vi "RealTimeAcq_SynthFoc_Rev1.vi"(4 "Frames/s":sgl=2.0, 5 "return to start":bool, 6 "Scan Axis":i8=3, 7 "Motion Board ID":T3=1 min=1 max=32 step=1, 8 "BKPT Shift":i32=75, 9 "mode":T1=enum."Full 25 Ch") -> (0 "error out":errorcluster, 2 "Bd ID Out":T2)   [LabVIEW 2022 SP3]
uses:
  ScanningControl/Motion Controllers/-MotionRoutines/MotionGlobals.vi
  <vilib>/Motion/FlexMotion/FunctionsVIs/Trajectory.llb/Load Acceleration/Deceleration.flx
  <vilib>/Motion/FlexMotion/CustomControls/CustomControls.llb/Axis To Control.flx
  <vilib>/Motion/FlexMotion/CustomControls/CustomControls.llb/Program.flx
  <instrlib>/niScope/Acquire/Fetch/niScope Multi Fetch Binary 8.vi
  <vilib>/Platform/TimedLoop/XDataNode/XDataNode.xnode
  <vilib>/Platform/TimedLoop/XDataNode/nitl_modes.ctl
  <vilib>/Platform/TimedLoop/XDataNode/XDNodeRunTimeDep.lvlib
  <vilib>/Platform/TimedLoop/XDataNode/wakeup.ctl
  <vilib>/Platform/TimedLoop/XDataNode/timing_clust.ctl
  <vilib>/Motion/FlexMotion/FunctionsVIs/Trajectory.llb/Wait for Move Complete (8 axes).flx
  <instrlib>/Acqiris Dx/Acqiris Dx.lvlib
  Annular Array/-SynthApperture/TimeShiftDataI8.vi
  <vilib>/DAQmx/write.llb/DAQmx Write (Digital 1D Bool NChan 1Samp 1Line).vi
  <vilib>/Analysis/NI_AALBase.lvlib
  <vilib>/Analysis/baseanly.llb/Mean (DBL).vi
  Real Time/-RT_support/RealTimeMode.ctl
panel:
  in  "Velocity Scale (%)":i16(slide) scale=50.0..110.0
  in  "Raw Name":string="raw"
  in  "Save Raw":bool
  in  "Type of Mean":u16(ring) items=["Mean from lines", "Mean just lines", "Poly Mean", "No mean"]
  out "Display queue":i32
  out "SF queue":i32
  out "Record queue":i32
  out "Display index":i32
  out "Read Loop":i32
  out "Read Data index":i32
  in  "Round to ROC?":bool
  in  "F3 20 MHz":dbl[](array[numeric])=[0.0, 0.0021173000000000003, 0.002217038688303391, 0.003063649156506908, 0.0031631091439381287, 0.0038030513383040436, 0.003902223261134889, 0.004435332245982045, 0.004534208485358321, 0.004999044189180914]
  in  "F2 40MHz":sgl[](array[numeric])=[0.0, 0.00132, 0.00142, 0.0019, 0.002, 0.00236, 0.00245, 0.00275, 0.00285, 0.0031]
  in  "One Way Receive":bool
  out "SF Index":i32
  in  "stop out":bool
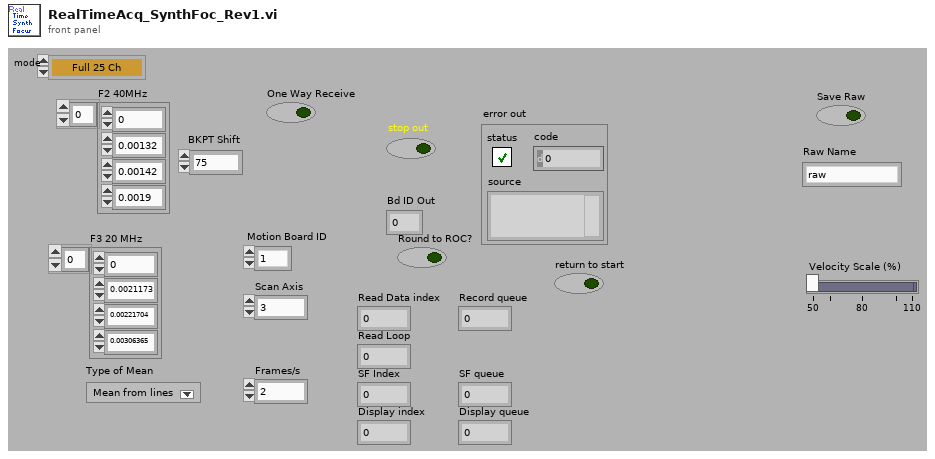
[diagram p1: front panel]
types:
  T1 = typedef "RealTimeMode.ctl" = enum16{"1T/5R", "1T/5R Deep Mem", "Full 25 Ch", "Drop Ch 5", "Drop Ch 5,4", "Drop Ch 5,4,3", "Drop Ch 5,4,3,2", "All 25 FIFO CH by CH", "Line by line 2 Ch", "Line by line All", "Deep Memory 2 CH", "Drop Ch 5 (3 Trig)", "test", "Drop Ch 5 XMIT", "Drop Ch 5,4 XMIT", "Drop Ch 5,4,3 XMIT"}
  T2 = typedef "Bd Id Out" = u8
  T3 = typedef "Board Id" = u8
  T4 = typedef "location.ctl" = enum16{"Automatic", "WCM Main", "Hawaii", "Columbia MM3000", "Columbia  NI System", "NYU", "RRI 2", "UHI Allen", "CUMC RT", "Chiba", "Stony Brook", "WCM Microscopy", "WCM Aeoretch", "WCM Optics Lab", "WCM Main 2Axis", "WCM Rotation", "WCM SAM SMAC", "SERI GP"}
  T5 = typedef "Program.flx" = u8
  T6 = typedef "XDNodeRunTimeDep.lvlib/timing_clust.ctl" = cluster{"Expected End [f-1]":u64, "Actual End [f-1]":u64, "Finished Late? [f-1]":bool, "Expected End [i-1]":u64, "Actual End [i-1]":u64, "Finished Late? [i-1]":bool, "Expected Start [i]":u64, "Actual Start [i]":u64, "Expected Start [f]":u64, "Actual Start [f]":u64, "Source Name":string, "Structure Name":string, "Period":i64, "Deadline":i64, "Offset":i64, "Start":i64, "Priority":i32, "Timeout":i32, "Mode":T7, "Wakeup Reason":T8, "Error":errorcluster, "Source Type":string, "Secondary Source Type":string, "Global End Time":u64, "Global Start Time":u64, "Frame Duration":u64, "Iteration Duration":u64, "Assigned CPU":i32, "I/O Scan Engine Mode":u32}
  T7 = typedef "XDNodeRunTimeDep.lvlib/nitl_modes.ctl" = enum32{"No Change", "Process missed periods, maintain original phase", "Discard missed periods, maintain original phase", "Process missed periods, ignore original phase", "Discard missed periods, ignore original phase"}
  T8 = typedef "XDNodeRunTimeDep.lvlib/wakeup.ctl" = enum32{"Normal", "Aborted", "Asynchronous wakeup", "Timing source error", "Timed loop error", "Timeout"}
  T9 = cluster{"gain":dbl, "wfm":i8[][], bool, "max queue size (-1, unlimited)":i32}
  T10 = typedef "Axis To Control.flx" = u16
  T11 = cluster{"ZoneStart":sgl[], "ZoneShift":sgl[], "ZoneLength":sgl[]}
  T12 = cluster{"ZoneStart":sgl[], "ZoneShift":sgl[], "ZoneLength":sgl[]}[][]
  T13 = cluster{"ZoneStart":sgl[], "ZoneShift":sgl[], "ZoneLength":sgl[]}[]
  T14 = cluster{"actualSamples":i32, "absoluteInitialX":dbl, "relativeInitialX":dbl, "xIncrement":dbl, "offset":dbl, "gain":dbl, "reserved1":dbl, "reserved2":dbl}[]
  T15 = cluster{"actualSamples":i32, "absoluteInitialX":dbl, "relativeInitialX":dbl, "xIncrement":dbl, "offset":dbl, "gain":dbl, "reserved1":dbl, "reserved2":dbl}
  T16 = cluster{"gain":dbl, "wfm":i8[][], "Reverse?":bool, i32}
  T17 = cluster{"dig gain":dbl, "Array":i8[][], "Reverse?":bool}
  T18 = typedef "Resource Out (Enum).flx" = u16
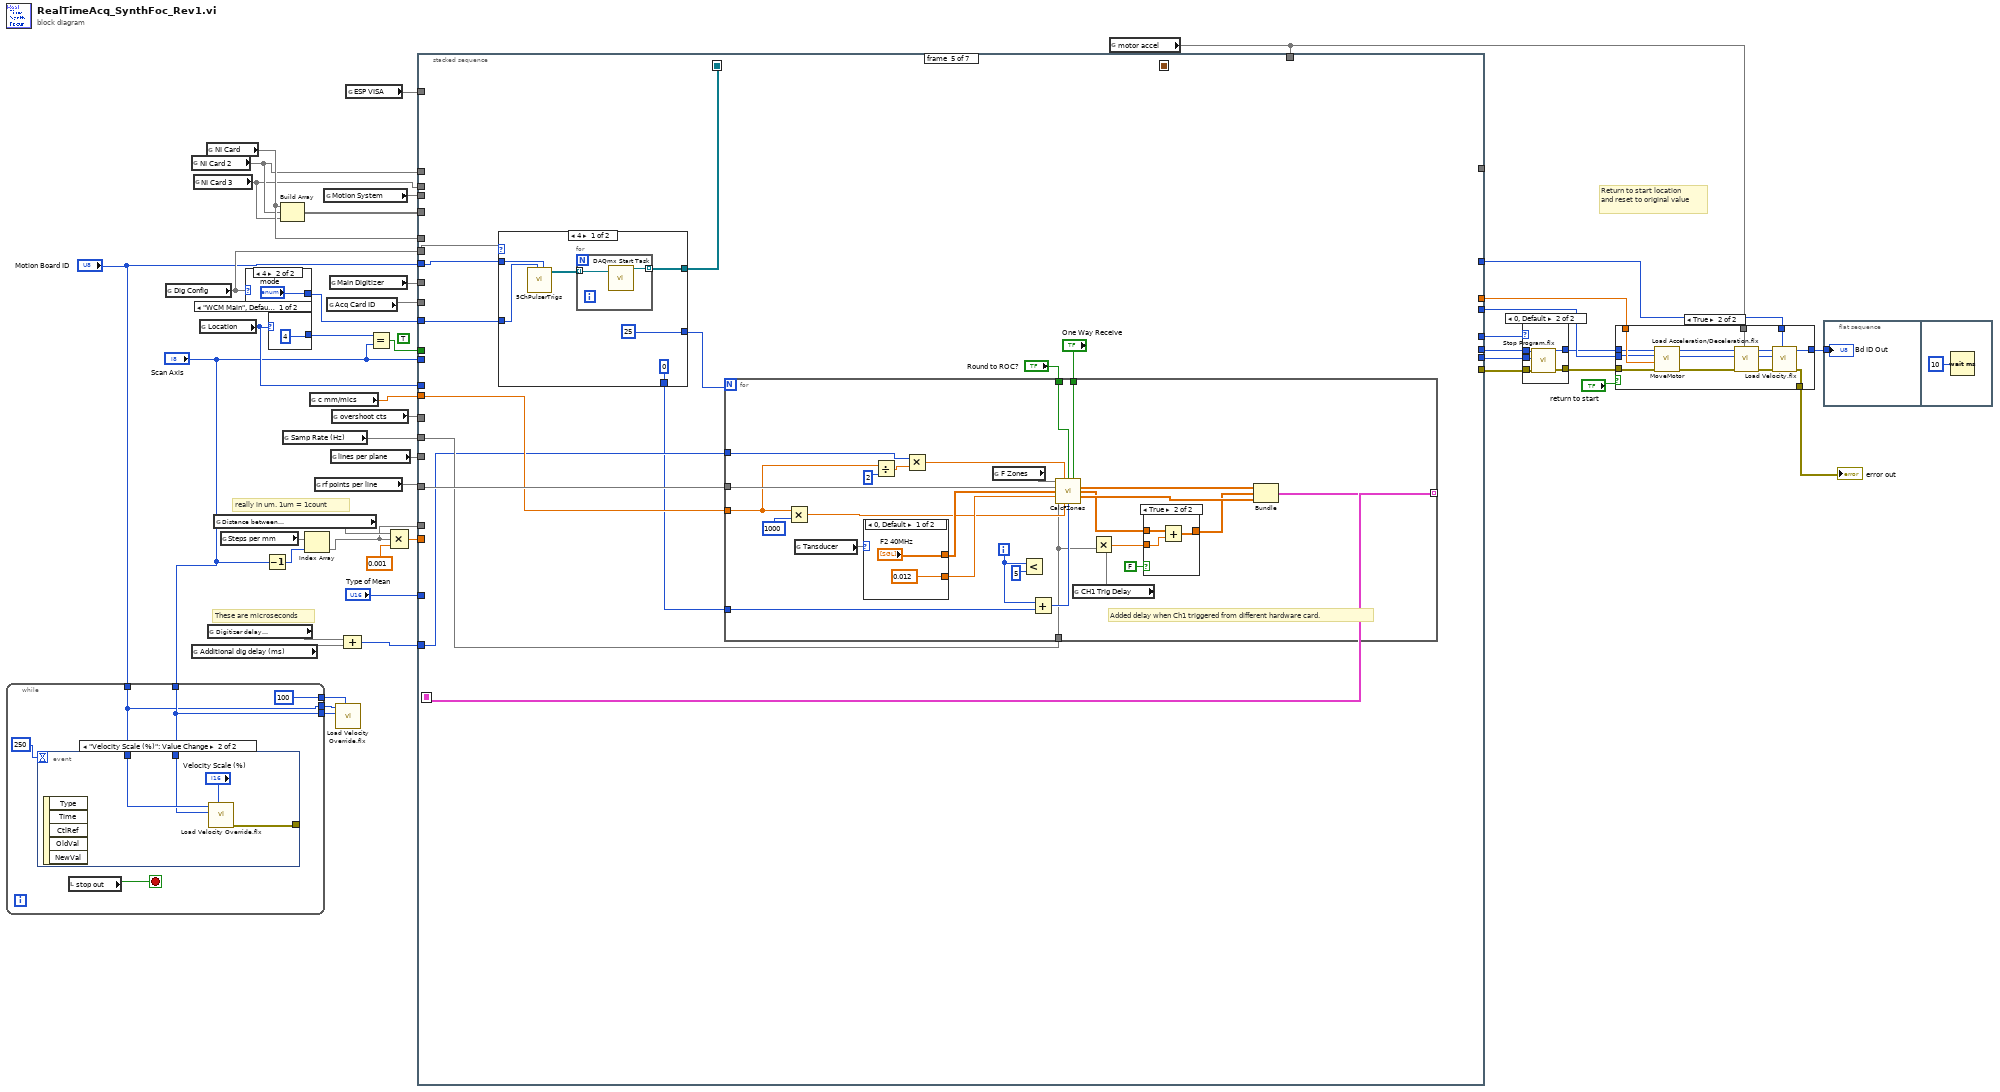
[diagram p0: block diagram]
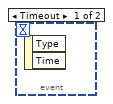
[diagram p2: hidden frame]
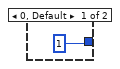
[diagram p3: hidden frame]
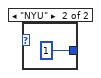
[diagram p6: hidden frame]
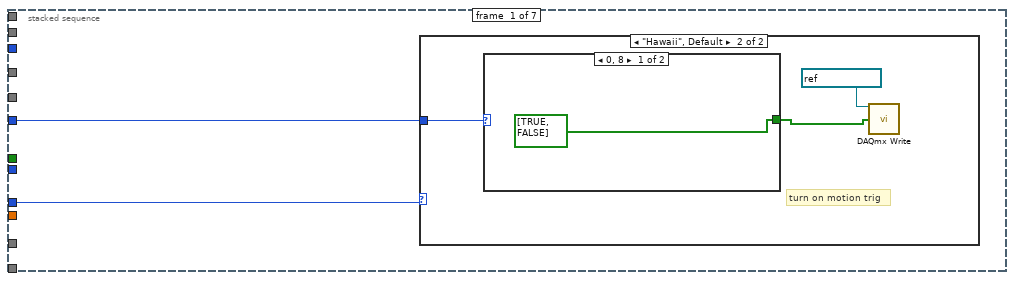
[diagram p7: hidden frame]
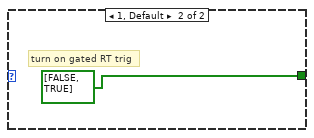
[diagram p9: hidden frame]
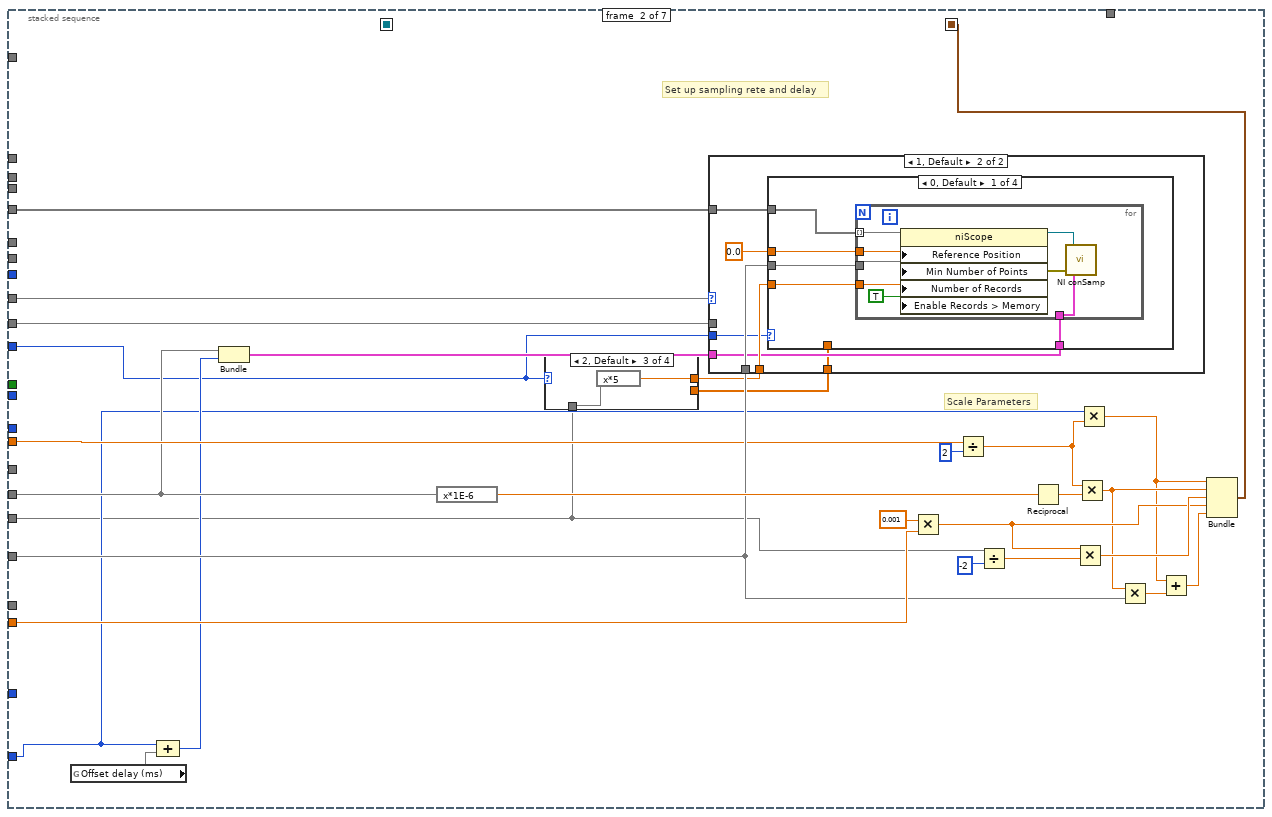
[diagram p10: hidden frame]
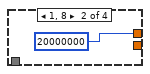
[diagram p12: hidden frame]
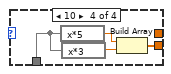
[diagram p13: hidden frame]
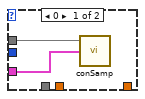
[diagram p14: hidden frame]
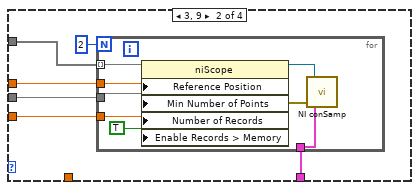
[diagram p15: hidden frame]
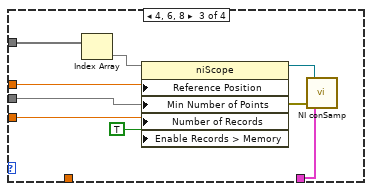
[diagram p16: hidden frame]
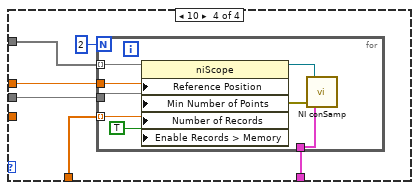
[diagram p17: hidden frame]
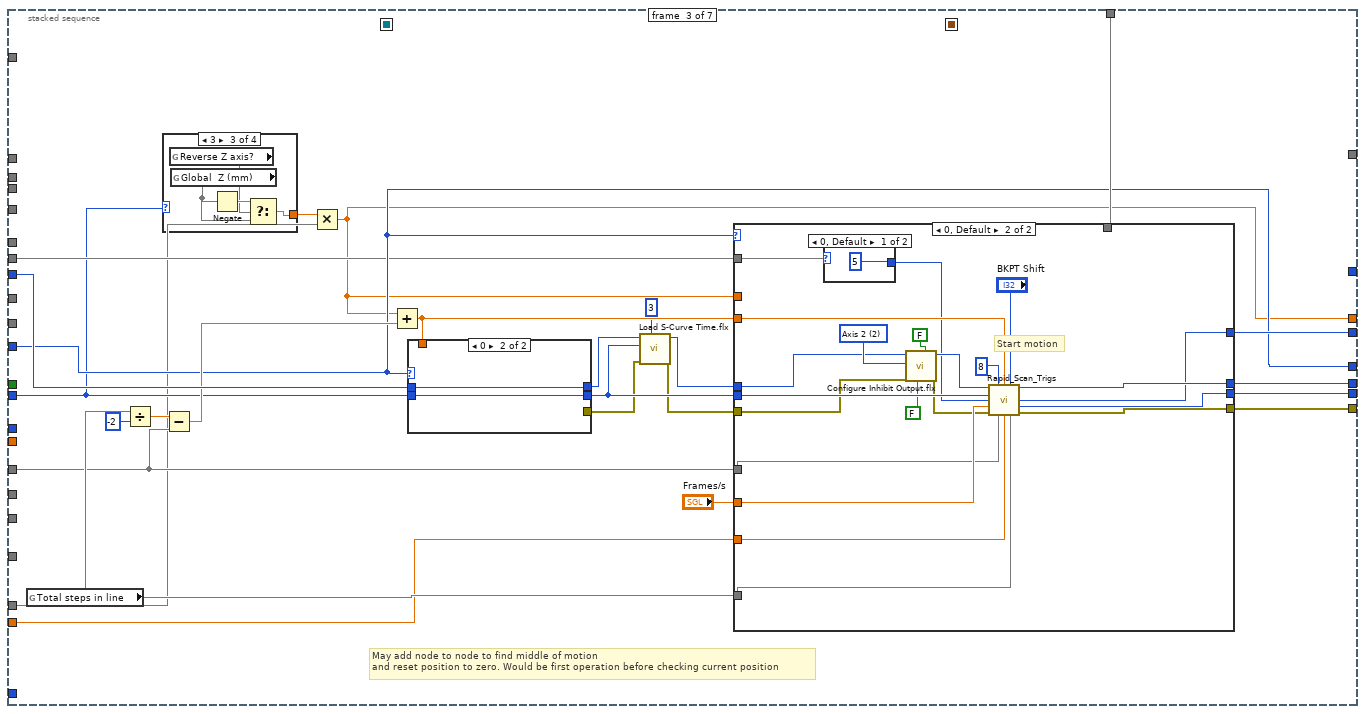
[diagram p18: hidden frame]
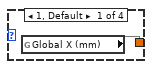
[diagram p19: hidden frame]
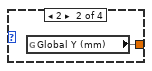
[diagram p20: hidden frame]
diagram:
  (unwired) TRUE
  # "These are microseconds"
  # "really in um. 1um = 1count"
  # "Return to start location and reset to original value"
  n1 = while {
    tunnel: "Motion Board ID" -> [w47]
    tunnel: "Scan Axis" -> [w48]
    tunnel: [100] -> w3
    tunnel: [w48] -> w2
    tunnel: [w47] -> w1
    stop <- w51 stop-if-true
    n2 = event shown="[1] \"Velocity Scale (%)\": Value Change" {
      selector: _ -> [_ _]
      dyn-events: _ -> [_ _]
      timeout: 250 -> [_ _]
      tunnel: w47 -> [_ w54]
      tunnel: w48 -> [_ w53]
      tunnel: [_ w52] -> _
      event Timeout {
        n3 = event-data() -> ()  [unwired: 1 in, 2 out]
      }
      event "Velocity Scale (%)": Value Change {
        n4 = event-data() -> ()  [unwired: 1 in, 5 out]
        n5 = call <vilib>:"Load Velocity Override.flx"("Override  Percentage (100%)"="Velocity Scale (%)", "Axis or Vector Space"=w53, "Board ID"=w54) -> ("error out"=w52:errorcluster)  [unwired: 4 in, 2 out]
      }
    }
    n6 = local read "stop out"() -> (w51:bool)
  }
  n7 = global read "MotionGlobals.vi" "Dig Config"() -> (w10)
  n8 = global read "MotionGlobals.vi" "NI Card 2"() -> (w14)
  n9 = global read "MotionGlobals.vi" "Additional dig delay (ms)"() -> (w25)
  n10 = global read "MotionGlobals.vi" "NI Card 3"() -> (w13)
  n11 = global read "MotionGlobals.vi" "Location"() -> (w28:T4)
  n12 = global read "MotionGlobals.vi" "NI Card"() -> (w15)
  n13 = global read "MotionGlobals.vi" "Digitizer delay\n (ms)"() -> (w26)
  n14 = global read "MotionGlobals.vi" "Distance between\nscan lines (mm)"() -> (w36)
  n15 = global read "MotionGlobals.vi" "Steps per mm"() -> (w9)
  n16 = case shown="4" w10 {
    tunnel: [i8 1 "mode"] -> w12
    frame 0, Default {
    }
    frame 4 {
    }
  }
  n17 = Decrement(x="Scan Axis") -> (x-1=w8:i8)
  n18 = case shown="\"WCM Main\", Default" w28 {
    tunnel: [i8 4 i8 1] -> w31
    frame "WCM Main", Default {
    }
    frame "NYU" {
    }
  }
  n19 = Build Array(w15, w14, w13) -> (w21:void[])
  n20 = global read "MotionGlobals.vi" "Samp Rate (Hz)"() -> (w23)
  n21 = Index Array(array=w9, index=w8) -> (element=w7)
  n22 = global read "MotionGlobals.vi" "c mm/mics"() -> (w27:sgl)
  n23 = global read "MotionGlobals.vi" "rf points per line"() -> (w45)
  n24 = global read "MotionGlobals.vi" "Motion System"() -> (w6)
  n25 = global read "MotionGlobals.vi" "Acq Card ID"() -> (w33)
  n26 = global read "MotionGlobals.vi" "Main Digitizer"() -> (w34)
  n27 = global read "MotionGlobals.vi" "lines per plane"() -> (w46)
  n28 = global read "MotionGlobals.vi" "overshoot cts"() -> (w44)
  n29 = call <vilib>:"Load Velocity Override.flx"("Override  Percentage (100%)"=w3, "Axis or Vector Space"=w2, "Board ID"=w1) -> ()  [unwired: 4 in, 3 out]
  n30 = Compound Arithmetic op=ADD(w26, w25) -> (w24:i32)
  n31 = global read "MotionGlobals.vi" "ESP VISA"() -> (w16)
  n32 = Equal?(x=w31, y="Scan Axis") -> (x = y?=w22:bool)
  n33 = Compound Arithmetic op=MULTIPLY(w36, w7, 0.001) -> (w35:dbl)
  n34 = global read "MotionGlobals.vi" "motor accel"() -> (w30)
  n35 = stacked-sequence {
    seq-local: [_ w87 _ _ _ _ _] -> [_ _ _ _ _ w312 _]
    seq-local: [_ _ _ _ w248 _ _] -> [_ _ _ _ _ w311 _]
    seq-local: [_ _ _ _ w245 _ _] -> [_ _ _ _ _ _ w2103]
    tunnel: w33 -> [_ w94 _ _ _ w320 _]
    tunnel: w46 -> [_ w69 _ _ _ w319 _]
    tunnel: [_ _ w187 _ _ _ _] -> w40
    tunnel: [_ _ w186 _ _ _ _] -> w42
    tunnel: w45 -> [_ w77 _ _ w254 w318 _]
    tunnel: [_ _ w184 _ _ _ _] -> w41
    tunnel: [_ _ w170 _ _ _ _] -> w39
    tunnel: w44 -> [_ _ w180 _ _ _ _]
    tunnel: [_ _ w183 _ _ _ _] -> w43
    tunnel: "Motion Board ID" -> [_ _ w179 w239 w244 w317 _]
    tunnel: [_ _ w174 _ _ _ _] -> w38
    tunnel: w12 -> [w60 w68 w174 _ w242 w307 w2104]
    tunnel: "Scan Axis" -> [_ _ w172 _ _ w308 _]
    tunnel: w35 -> [_ w80 w178 _ _ _ _]
    tunnel: w34 -> [_ w79 _ _ _ w316 _]
    tunnel: w15 -> [_ _ _ _ _ w315 _]
    tunnel: [_ _ _ _ _ w314 _] -> w32
    tunnel: w30 -> [_ _ w176 _ _ _ _]
    tunnel: w6 -> [_ _ _ w240 _ w313 _]
    tunnel: [_ _ _ _ _ w313 _] -> _
    tunnel: w28 -> [w61 _ _ _ _ w309 w2106]
    tunnel: w27 -> [_ w76 _ _ w253 _ _]
    tunnel: w24 -> [_ w72 _ _ w251 _ _]
    tunnel: w23 -> [_ w75 _ _ w252 _ _]
    tunnel: w22 -> [_ _ _ _ _ w306 _]
    tunnel: w21 -> [_ w71 _ _ _ w310 _]
    tunnel: w16 -> [_ _ _ _ _ _ _]
    tunnel: w14 -> [_ _ _ _ _ w305 _]
    tunnel: w13 -> [_ _ _ _ _ w304 _]
    tunnel: "Type of Mean" -> [_ _ _ _ _ w303 _]
    tunnel: w10 -> [_ _ w173 _ w243 _ _]
    tunnel: w7 -> [_ _ w169 _ _ _ _]
    frame #0 {
      n36 = case shown="\"Hawaii\", Default" w61 {
        tunnel: w60 -> [_ w64]
        frame "UHI Allen" {
        }
        frame "Hawaii", Default {
          # "turn on motion trig"
          n37 = case shown="0, 8" w64 {
            tunnel: [bool[] [TRUE, FALSE] ("data") bool[] [FALSE, TRUE] ("data")] -> w62
            frame 0, 8 {
            }
            frame 1, Default {
              # "turn on gated RT trig"
            }
          }
          n38 = call-poly <vilib>:"DAQmx Write.vi"("task/channels in"=refnum<k21> "DIO-L2 L3", "data"=w62) -> ()  [unwired: 11 in, 3 out]
        }
      }
    }
    frame #1 {
      # "Scale Parameters"
      # "Set up sampling rete and delay"
      n39 = global read "MotionGlobals.vi" "Offset delay (ms)"() -> (w74)
      n40 = Compound Arithmetic op=ADD(w72, w74) -> (w73:i32)
      n41 = Bundle("Samp Rate (Hz)"=w75, w73) -> (w95:cluster{"Samp Rate (Hz)":void, i32})  [unwired: 1 out]
      n42 = expression code="x*1E-6"(w75) -> (w78:dbl)
      n43 = case shown="2, Default" w68 {
        tunnel: [w96 20000000 w98 _] -> w70
        tunnel: w69 -> [w96 _ w99 w103]
        tunnel: [_ _ _ w100] -> w67
        frame 0 {
        }
        frame 1, 8 {
        }
        frame 2, Default {
          n44 = expression code="x*5"(w99) -> (w98:dbl)
        }
        frame 10 {
          n45 = expression code="x*5"(w103) -> (w102:dbl)
          n46 = expression code="x*3"(w103) -> (w101:dbl)
          n47 = Build Array(w102, w101) -> (w100:dbl[])
        }
      }
      n48 = case shown="1, Default" w79 {
        tunnel: w95 -> [w105 w110]
        tunnel: w94 -> [w104 _]
        tunnel: w77 -> [_ w111]
        tunnel: w70 -> [_ w112]
        tunnel: w71 -> [_ w109]
        tunnel: w68 -> [_ w107]
        tunnel: w67 -> [_ w106]
        frame 0 {
          n49 = call "conSamp.vi"("Sampling"=w105, "InstrumentID"=w104) -> ()  [unwired: 1 in, 2 out]
        }
        frame 1, Default {
          n50 = case shown="0, Default" w107 {
            tunnel: w112 -> [w117 w131 w148 _]
            tunnel: w111 -> [w116 w130 w147 w154]
            tunnel: w110 -> [w115 w129 w146 w153]
            tunnel: w109 -> [w114 w128 w144 w152]
            tunnel: 0.0 -> [w113 w127 w145 w151]
            tunnel: w106 -> [_ _ _ w149]
            frame 0, Default {
              n51 = for {
                tunnel: w117 -> [w120]
                tunnel: w116 -> [w125]
                tunnel: w114 -> [w122] mode=indexing
                tunnel: w115 -> [w121]
                tunnel: w113 -> [w119]
                n52 = property class="niScope"(reference=w122, "Reference Position"=w119, "Min Number of Points"=w125, "Number of Records"=w120, "Enable Records > Memory"=TRUE) -> (reference out=w124:refnum<k15>, error out=w123:errorcluster)  [unwired: 1 in]
                n53 = call "NI conSamp.vi"("error in"=w123, "Sampling"=w121, "InstrumentID"=w124) -> ()  [unwired: 2 out]
              }
            }
            frame 3, 9 {
              n54 = for {
                N: 2 -> [_]
                tunnel: w131 -> [w134]
                tunnel: w130 -> [w139]
                tunnel: w128 -> [w136] mode=indexing
                tunnel: w129 -> [w135]
                tunnel: w127 -> [w133]
                n55 = property class="niScope"(reference=w136, "Reference Position"=w133, "Min Number of Points"=w139, "Number of Records"=w134, "Enable Records > Memory"=TRUE) -> (reference out=w138:refnum<k15>, error out=w137:errorcluster)  [unwired: 1 in]
                n56 = call "NI conSamp.vi"("error in"=w137, "Sampling"=w135, "InstrumentID"=w138) -> ()  [unwired: 2 out]
              }
            }
            frame 4, 6, 8 {
              n57 = Index Array(array=w144) -> (element=w140)  [unwired: 1 in]
              n58 = property class="niScope"(reference=w140, "Reference Position"=w145, "Min Number of Points"=w147, "Number of Records"=w148, "Enable Records > Memory"=TRUE) -> (reference out=w143:refnum<k15>, error out=w142:errorcluster)  [unwired: 1 in]
              n59 = call "NI conSamp.vi"("error in"=w142, "Sampling"=w146, "InstrumentID"=w143) -> ()  [unwired: 2 out]
            }
            frame 10 {
              n60 = for {
                N: 2 -> [_]
                tunnel: w149 -> [w157] mode=indexing
                tunnel: w154 -> [w162]
                tunnel: w152 -> [w159] mode=indexing
                tunnel: w153 -> [w158]
                tunnel: w151 -> [w156]
                n61 = property class="niScope"(reference=w159, "Reference Position"=w156, "Min Number of Points"=w162, "Number of Records"=w157, "Enable Records > Memory"=TRUE) -> (reference out=w161:refnum<k15>, error out=w160:errorcluster)  [unwired: 1 in]
                n62 = call "NI conSamp.vi"("error in"=w160, "Sampling"=w158, "InstrumentID"=w161) -> ()  [unwired: 2 out]
              }
            }
          }
        }
      }
      n63 = Multiply(x=0.001, y=w80) -> (x*y=w85:dbl)
      n64 = Divide(x=w76, y=2) -> (x/y=w88:sgl)
      n65 = Divide(x=w69, y=-2) -> (x/y=w90:dbl)
      n66 = Reciprocal(x=w78) -> (1/x=w93:dbl)
      n67 = Multiply(x=w85, y=w90) -> (x*y=w86:dbl)
      n68 = Multiply(x=w88, y=w93) -> (x*y=w84:dbl)
      n69 = Multiply(x=w72, y=w88) -> (x*y=w82:sgl)
      n70 = Multiply(x=w84, y=w77) -> (x*y=w83:dbl)
      n71 = Add(x=w82, y=w83) -> (x+y=w81:sgl)
      n72 = Bundle(w82, w84, w86, w85, w81) -> (w87:cluster{sgl, dbl, dbl, dbl, sgl})  [unwired: 1 out]
    }
    frame #2 {
      # "May add node to node to find middle of motion\nand reset position to zero. Would be first operation before checking current position"
      n73 = global read "MotionGlobals.vi" "Total steps in line"() -> (w182)
      n74 = Divide(x=w182, y=-2) -> (x/y=w181:dbl)
      n75 = case shown="3" w172 {
        tunnel: [w189 w190 w191 w195] -> w171
        frame 1, Default {
          n76 = global read "MotionGlobals.vi" "Global X (mm)"() -> (w189)
        }
        frame 2 {
          n77 = global read "MotionGlobals.vi" "Global Y (mm)"() -> (w190)
        }
        frame 3 {
          n78 = global read "MotionGlobals.vi" "Reverse Z axis?"() -> (w192)
          n79 = global read "MotionGlobals.vi" "Global  Z (mm)"() -> (w193)
          n80 = Negate(x=w193) -> (-x=w194:dbl)
          n81 = Select(t=w194, s=w192, f=w193) -> (s? t:f=w191:dbl)
        }
        frame 4 {
          n82 = global read "MotionGlobals.vi" "Global  Axis 4"() -> (w195)
        }
      }
      n83 = Subtract(x=w181, y=w180) -> (x-y=w177:dbl)
      n84 = Multiply(x=w171, y=w169) -> (x*y=w170:dbl)
      n85 = Add(x=w170, y=w177) -> (x+y=w175:dbl)
      n86 = case shown="0" w174 {
        tunnel: w179 -> [w201 w203]
        tunnel: w172 -> [w200 w202]
        tunnel: [w199 w203] -> w168
        tunnel: [w198 w202] -> w166
        tunnel: [w197 _] -> w164
        tunnel: w175 -> [w196 _]
        frame 1, Default {
          n87 = call "MoveMotor.vi"("Target Position (0)"=w196, "Axis or Vector Space"=w200, "Motion Bd ID"=w201) -> ("error out"=w197:errorcluster, "Resource Output"=w198:u16, "Bd ID Out"=w199:u8)  [unwired: 2 in, 4 out]
        }
        frame 0 {
        }
      }
      n88 = call <vilib>:"Load S-Curve Time.flx"("S Curve Time (1)"=u16 3, "error in (no error)"=w164, "Axis or Vector Space"=w166, "Board ID"=w168) -> ("error out"=w163:errorcluster, "Bd ID Out"=w167:T2)  [unwired: 3 in, 1 out]
      n89 = case shown="0, Default" w174 {
        tunnel: "Frames/s" -> [w213 w236]
        tunnel: [w204 w235] -> w187
        tunnel: [w215 w234] -> w186
        tunnel: [_ w233] -> w184
        tunnel: [w214 w232] -> w183
        tunnel: w182 -> [w211 w231]
        tunnel: w178 -> [_ w230]
        tunnel: w180 -> [_ w229]
        tunnel: w167 -> [w215 w219]
        tunnel: w166 -> [w214 w228]
        tunnel: w163 -> [w205 w218]
        tunnel: w175 -> [_ w227]
        tunnel: w170 -> [w212 _]
        tunnel: w176 -> [_ _]
        tunnel: w173 -> [_ w216]
        frame 1, 8 {
          w207 = T5 6 ("Program (1)")
          w210 = FALSE
          n90 = call "Modulo_Triggers.vi"("Motion Settings In"=w215, "Axis"=w214, "Reverse ?"=w210, "Program (1)"=w207, 7:w213, "error in (no error)"=w205, 12:w211, "Offset"=w212) -> ("error out"=w206:errorcluster)  [unwired: 1 in, 6 out]
          n91 = Increment(x=w207) -> (x+1=w208:T5)
          n92 = Not(x=w210) -> (.not. x?=w209:bool)
          n93 = call "Modulo_Triggers.vi"("Motion Settings In"=w215, "Axis"=w214, "Reverse ?"=w209, "Program (1)"=w208, 7:w213, "error in (no error)"=w206, 12:w211, "Offset"=w212) -> ("error out"=w204:errorcluster)  [unwired: 1 in, 6 out]
        }
        frame 0, Default {
          w222 = T10 2 items=["Axis 1"=1, "Axis 2"=2, "Axis 3"=3, "Axis 4"=4, "Axis 5"=5, "Axis 6"=6, "Axis 7"=7, "Axis 8"=8] ("Axis")
          # "Start motion"
          n94 = case shown="0, Default" w216 {
            tunnel: [u32 5 u32 5 ("EOL Delay (ms)")] -> w217
            frame 0, Default {
            }
            frame 2 {
            }
          }
          n95 = call <vilib>:"Configure Inhibit Output.flx"("Enable"=FALSE, "Polarity (Active Low)"=FALSE, "error in (no error)"=w218, "Axis"=w222, "Board ID"=w219) -> ("error out"=w225:errorcluster, "Bd ID Out"=w226:T2)  [unwired: 1 in, 4 out]
          n96 = call "Rapid_Scan_Trigs.vi"("Board ID"=w226, "Program (1)"=T5 8, "Start Position"=w227, "BKPT Shift"="BKPT Shift", "Scan Axis"=w228, "Pause?"=w217, "# frames/ s"=w236, "error in (no error)"=w225, "overshoot"=w229, "step interval"=w230, "Total Steps (one way)"=w231) -> ("Bd ID Out"=w234:u8, "Axis Resource out"=w232:u16, "Program ID"=w233:u8, "error out"=w235:errorcluster)  [unwired: 1 out]
        }
      }
    }
    frame #3 {
      n97 = case shown="0, Default" w240 {
        tunnel: w239 -> [w241 _]
        frame 0, Default {
          n98 = call "CheckLimStat.vi"("Motion Board ID"=w241) -> ()
        }
        frame 1, 7 {
        }
      }
    }
    frame #4 {
      n99 = case shown="4" w243 {
        tunnel: [25 5] -> w247
        tunnel: [u32 0 w263] -> w246
        tunnel: [w257 _] -> w245
        tunnel: w244 -> [w256 _]
        tunnel: w242 -> [w255 _]
        frame 4 {
          n100 = call "5ChPulserTrigs.vi"("Motion Board ID"=w256, "mode"=w255) -> ("5CH Pulser Tasks"=w258:refnum<k21>[])  [unwired: 7 in, 1 out]
          n101 = for {
            tunnel: w258 -> [w262] mode=indexing
            tunnel: [w261] -> w257 mode=indexing
            n102 = call <vilib>:"DAQmx Start Task.vi"("task/channels in"=w262) -> ("task out"=w261:refnum<k21>)  [unwired: 13 in, 1 out]
          }
        }
        frame 0, Default {
          n103 = global read "MotionGlobals.vi" "Switch T/R"() -> (w266)
          n104 = Decrement(x=w266) -> (x-1=w265:dbl)
          n105 = Multiply(x=w265, y=5) -> (x*y=w263:i32)
        }
      }
      n106 = for {
        N: w247 -> [_]
        tunnel: w254 -> [w287]
        tunnel: w253 -> [w280]
        tunnel: w252 -> [w274]
        tunnel: w251 -> [w286]
        tunnel: "One Way Receive" -> [w285]
        tunnel: "Round to ROC?" -> [w284]
        tunnel: [w282] -> w248 mode=indexing
        tunnel: w246 -> [w277]
        i -> [w276]
        # "Added delay when Ch1 triggered from different hardware card."
        n107 = Multiply(x=w280, y=1000) -> (x*y=w281:sgl)
        n108 = global read "MotionGlobals.vi" "Tansducer"() -> (w290)
        n109 = case shown="0, Default" w290 {
          tunnel: ["F2 40MHz" "F3 20 MHz"] -> w289
          tunnel: [0.012 ("ROC (mm)") 0.031 ("ROC (mm)")] -> w288
          frame 0, Default {
          }
          frame 1 {
          }
        }
        n110 = Divide(x=w280, y=2) -> (x/y=w293:sgl)
        n111 = Multiply(x=w286, y=w293) -> (x*y=w279:sgl)
        n112 = global read "MotionGlobals.vi" "F Zones"() -> (w292)
        n113 = Less?(x=w276, y=5) -> ()  [unwired: 1 out]
        n114 = Add(x=w276, y=w277) -> (x+y=w278:u32)
        n115 = call "CalcFZones.vi"("F- zones"=w292, "delay (mm)"=w279, "Round to ROC?"=w284, "One Way Receive"=w285, "# rf points per line"=w287, "Radii (m)"=w289, "ROC (m)"=w288, "Sampling Rate"=w274, "c (m/s)"=w281, "File index number"=w278) -> ("ZoneStart"=w272:sgl[], "ZoneShift"=w271:sgl[], "ZoneLength"=w283:sgl[])  [unwired: 3 out]
        n116 = global read "MotionGlobals.vi" "CH1 Trig Delay"() -> (w269)
        n117 = Multiply(x=w269, y=w274) -> (x*y=w273:dbl)
        n118 = case shown="True" FALSE {
          tunnel: w271 -> [w295 w297]
          tunnel: [w295 w298] -> w270
          tunnel: w273 -> [_ w296]
          frame False {
          }
          frame True {
            n119 = Add(x=w297, y=w296) -> (x+y=w298:sgl[])
          }
        }
        n120 = Bundle("ZoneStart"=w272, "ZoneShift"=w270, "ZoneLength"=w283) -> (w282:T11)  [unwired: 1 in]
      }
    }
    frame #5 {
      n121 = case shown="True" w306 {
        tunnel: w320 -> [w328 _]
        tunnel: w319 -> [w329 w424]
        tunnel: w318 -> [w330 w423]
        tunnel: w317 -> [w326 w425]
        tunnel: w312 -> [w325 w422]
        tunnel: w316 -> [w324 _]
        tunnel: w315 -> [w323 w417]
        tunnel: [w322 w426] -> w314
        tunnel: w313 -> [w321 _]
        tunnel: w311 -> [_ w421]
        tunnel: w307 -> [_ w420]
        tunnel: w310 -> [_ w419]
        tunnel: w309 -> [_ _]
        tunnel: w308 -> [_ w418]
        tunnel: w305 -> [_ w416]
        tunnel: w304 -> [_ w415]
        tunnel: w303 -> [_ w414]
        frame False {
          n122 = while {
            tunnel: w330 -> [w352]
            tunnel: w329 -> [w342]
            tunnel: w328 -> [w351]
            shift-right: [w350] -> _
            shift-left: TRUE -> [w334]
            tunnel: w326 -> [w349]
            tunnel: w325 -> [w345]
            tunnel: w324 -> [w343]
            tunnel: w323 -> [w341]
            tunnel: w321 -> [w335]
            i -> [w344]
            stop <- w348 stop-if-true
            # "Display data"
            # "Get data"
            # "This is slower version for heavier mass motors. Scan stop, read data, scan etc"
            n123 = Select(t="1", s=w334, f="2") -> (s? t:f=w331:string)
            n124 = Select(t=T5 6 ("Program (1)"), s=w334, f=T5 7 ("Program (1)")) -> (s? t:f=w338:T5)
            n125 = case shown="1, Default" w343 {
              tunnel: w352 -> [w362 w390]
              tunnel: w342 -> [w361 w389]
              tunnel: w351 -> [w375 _]
              tunnel: w349 -> [w374 w401]
              tunnel: [w373 w400] -> w347
              tunnel: w338 -> [w369 w399]
              tunnel: [w356 w391] -> w340
              tunnel: w341 -> [_ w393]
              tunnel: w334 -> [w358 w384]
              tunnel: [w359 w383] -> w339
              tunnel: w335 -> [_ _]
              tunnel: w331 -> [_ _]
              frame 0 {
                n126 = call <instrlib>:"Configure Memory Settings.vi"("Number of Samples (1000)"=w362, "Number of Segments (1)"=w361, "Instrument ID"=w375) -> ("error out"=w372:errorcluster, "dup Instrument ID"=w370:u32)  [unwired: 1 in, 2 out]
                n127 = call <instrlib>:"Start Acquisition.vi"("error in (no error)"=w372, "Instrument ID"=w370) -> ("error out"=w368:errorcluster, "dup Instrument ID"=w371:u32)  [unwired: 2 in]
                n128 = stacked-sequence {
                  tunnel: w368 -> [w382]
                  tunnel: [w382] -> w367
                  frame #0 {
                    n129 = Wait (ms)(milliseconds to wait=20) -> ()  [unwired: 1 out]
                  }
                }
                n130 = call <vilib>:"Run Program.flx"("error in (no error)"=w367, "Program (1)"=w369, "Board ID"=w374) -> ("error out"=w366:errorcluster, "Bd ID Out"=w373:T2)  [unwired: 4 out]
                n131 = stacked-sequence {
                  tunnel: w366 -> [w379]
                  tunnel: [w379] -> w365
                  frame #0 {
                    n132 = Wait (ms)(milliseconds to wait=20) -> ()  [unwired: 1 out]
                  }
                }
                n133 = call "WaitForSegs.vi"("Acqiris ID"=w371, "lines per plane"=w361, "error in"=w365, "Timeout"=5000) -> ("dup Instrument ID"=w364:u32, "error out"=w363:errorcluster)  [unwired: 2 out]
                n134 = call "GetWaveform.vi"("Acq ID Out"=w364, "Num Samps"=w362, "Num Segs"=w361, "error in"=w363) -> ("Acquired Waveform16 bit"=w360:i16[][], "error out"=w356:errorcluster)  [unwired: 2 in, 8 out]
                n135 = case shown="True" w358 {
                  tunnel: w360 -> [w376 w378]
                  tunnel: [w376 w377] -> w359
                  frame False {
                  }
                  frame True {
                    n136 = call "ReverseData.vi"("Array in"=w378) -> ("Array out"=w377:i16[][])
                  }
                }
              }
              frame 1, Default {
                w387 = u16 1 items=["Simple Read", "RT Read", "RT Save", "Scaled Voltage"] ("Read Method")
                n137 = property class="niScope"(reference=w393, "Number of Records"=w389, "Min Number of Points"=w390) -> (reference out=w395:refnum<k15>, error out=w394:errorcluster)  [unwired: 1 in]
                n138 = call <instrlib>:"niScope Initiate Acquisition.vi"("instrument handle"=w395, "error in"=w394) -> ("instrument handle out"=w388:refnum<k15>, "error out"=w398:errorcluster)  [unwired: 1 in, 11 out]
                n139 = stacked-sequence {
                  tunnel: w398 -> [w405]
                  tunnel: [w405] -> w397
                  frame #0 {
                    n140 = Wait (ms)(milliseconds to wait=u32 5) -> ()  [unwired: 1 out]
                  }
                }
                n141 = call <vilib>:"Run Program.flx"("error in (no error)"=w397, "Program (1)"=w399, "Board ID"=w401) -> ("error out"=w396:errorcluster, "Bd ID Out"=w400:T2)  [unwired: 4 out]
                n142 = stacked-sequence {
                  tunnel: w396 -> [w402]
                  tunnel: [w402] -> w392
                  frame #0 {
                    n143 = Wait (ms)(milliseconds to wait=u32 20) -> ()  [unwired: 1 out]
                  }
                }
                n144 = call "NI GetWaveform.vi"("Acq ID In"=w388, "Read Method"=w387, "timeout"=5.0, "Num Samps"=w390, "Reverse?"=w384, "Num Segs"=w389, "error in"=w392, "Channel"=1) -> ("Acquired Waveform16 bit"=w383:i8[][], "error out"=w391:errorcluster)  [unwired: 2 in, 4 out]
              }
            }
            n145 = case shown="No Error" w340 {
              selector: w340 -> [w407 w412]
              tunnel: [w408 w412] -> w346
              tunnel: [w411 TRUE] -> w348
              tunnel: w345 -> [w410 _]
              tunnel: w344 -> [w409 _]
              tunnel: w339 -> [w406 _]
              frame No Error {
                n146 = call "CurrentPlane.vi"("Axis Vals"=w410, "error in"=w407, "Frame"=w409, "Data"=w406) -> ("error out"=w408:errorcluster, "stop out"=w411:bool)  [unwired: 6 in]
              }
              frame Error {
              }
            }
            n147 = local write "SF Index"(w344) -> ()
            n148 = case shown="1, Default" w335 {
              tunnel: w347 -> [_ w355]
              tunnel: w346 -> [_ w354]
              tunnel: w338 -> [_ w353]
              frame 7 {
              }
              frame 1, Default {
                n149 = call <vilib>:"Stop Program.flx"("error in (no error)"=w354, "Program (1)"=w353, "Board ID"=w355) -> ()  [unwired: 6 out]
              }
            }
            n150 = Not(x=w334) -> (.not. x?=w350:bool)
          }
          n151 = global read "MotionGlobals.vi" "motor velocity"() -> (w322)
        }
        frame True {
          n152 = case shown="2" w420 {
            tunnel: [40000 40000 40000 40000 40000 40000 40000 40000 40000 40000 40000] -> w426
            tunnel: w425 -> [w452 w603 w757 w945 w1115 w1225 w1391 w1476 w1593 w1760 w1945]
            tunnel: w424 -> [w451 w599 w761 w927 w1111 w1229 w1392 w1477 w1558 w1742 w1921]
            tunnel: w423 -> [w450 w600 w738 w929 w1101 w1221 w1378 w1490 w1561 w1744 w1929]
            tunnel: w422 -> [w429 w568 w763 w950 w1120 w1231 w1397 w1484 w1578 w1765 w1950]
            tunnel: w421 -> [w445 w594 w771 w958 w1128 w1240 w1382 w1478 w1567 w1773 w1958]
            tunnel: w419 -> [w438 w577 _ _ _ _ _ w1471 _ _ _]
            tunnel: w418 -> [_ w579 _ _ _ _ _ _ w1586 _ _]
            tunnel: w417 -> [_ _ w749 w926 w1106 w1222 w1379 _ w1582 w1741 w1927]
            tunnel: w416 -> [_ _ w774 w924 _ w1243 _ _ _ w1739 w1925]
            tunnel: w415 -> [_ _ w773 _ _ w1242 _ _ _ _ _]
            tunnel: w414 -> [_ _ _ _ _ _ _ _ _ _ _]
            frame 0, Default {
              # "1T/5R flip flop version"
              n153 = Array To Cluster(array=w438) -> (cluster=w437:cluster{"[0]":void, "[1]":void, "[2]":void})
              n154 = Unbundle(w437) -> ("[0]"=w428, "[1]"=w436, "[2]"=w435)
              n155 = Obtain Queue(max queue size (-1, unlimited)=4, element data type=cluster{"gain":dbl, bool} {"gain"=0.0, TRUE}) -> (queue out=w460:refnum<queue>)  [unwired: 2 in, 3 out]
              n156 = Index Array(array=w445) -> (element=w442:T11)  [unwired: 1 in]
              n157 = Index Array(array=w445, index=1) -> (element=w441:T11)
              n158 = Index Array(array=w445, index=2) -> (element=w440:T11)
              n159 = Index Array(array=w445, index=3) -> (element=w443:T11)
              n160 = Index Array(array=w445, index=4) -> (element=w444:T11)
              n161 = Obtain Queue(max queue size (-1, unlimited)=20, element data type=i8[][] [] ("Array")) -> (queue out=w453:refnum<queue>)  [unwired: 2 in, 3 out]
              n162 = Obtain Queue(max queue size (-1, unlimited)=4, element data type=cluster{bool, "Array":i16[][]} {TRUE, "Array"=[]}) -> (queue out=w433:refnum<queue>)  [unwired: 3 in, 2 out]
              n163 = while {
                tunnel: w460 -> [w489]
                tunnel: [w520] -> w458
                tunnel: [w498] -> w457
                tunnel: w453 -> [w490]
                tunnel: w444 -> [w511]
                tunnel: w443 -> [w510]
                tunnel: w442 -> [w509]
                tunnel: w441 -> [w508]
                tunnel: w440 -> [w507]
                tunnel: [w485] -> w439
                tunnel: w433 -> [w502]
                i -> [w499]
                stop <- w520 stop-if-true
                w495 = 5000 ("timeout in ms (-1)")
                # "Dequeue data and synth focus"
                n164 = Dequeue Element(queue=w489, timeout in ms (-1)=w495) -> (queue out=w498:refnum<queue>, element=w519:cluster{"gain":dbl, bool}, error out=w497:errorcluster)  [unwired: 1 in, 1 out]
                n165 = Dequeue Element(queue=w490, timeout in ms (-1)=w495, error in (no error)=w497) -> (queue out=w488:refnum<queue>, element=w496:i8[][], error out=w494:errorcluster)  [unwired: 1 out]
                n166 = Unbundle(w519) -> (w501:bool)  [unwired: 1 out]
                n167 = call-poly "TimeShiftDataPoly.vi"("output cluster"=w509, "Array In"=w496) -> ("Array Out"=w482:i8[][])  [unwired: 1 in, 1 out]
                n168 = Dequeue Element(queue=w488, timeout in ms (-1)=w495, error in (no error)=w494) -> (queue out=w518:refnum<queue>, element=w515:i8[][], error out=w493:errorcluster)  [unwired: 1 out]
                n169 = call-poly "TimeShiftDataPoly.vi"("output cluster"=w508, "Array In"=w515) -> ("Array Out"=w506:i8[][])  [unwired: 1 in, 1 out]
                n170 = Dequeue Element(queue=w518, timeout in ms (-1)=w495, error in (no error)=w493) -> (queue out=w517:refnum<queue>, element=w514:i8[][], error out=w492:errorcluster)  [unwired: 1 out]
                n171 = call-poly "TimeShiftDataPoly.vi"("output cluster"=w507, "Array In"=w514) -> ("Array Out"=w505:i8[][])  [unwired: 1 in, 1 out]
                n172 = Dequeue Element(queue=w517, timeout in ms (-1)=w495, error in (no error)=w492) -> (queue out=w516:refnum<queue>, element=w513:i8[][], error out=w491:errorcluster)  [unwired: 1 out]
                n173 = call-poly "TimeShiftDataPoly.vi"("output cluster"=w510, "Array In"=w513) -> ("Array Out"=w504:i8[][])  [unwired: 1 in, 1 out]
                n174 = Dequeue Element(queue=w516, timeout in ms (-1)=w495, error in (no error)=w491) -> (queue out=w486:refnum<queue>, element=w512:i8[][], error out=w487:errorcluster)  [unwired: 1 out]
                n175 = call-poly "TimeShiftDataPoly.vi"("output cluster"=w511, "Array In"=w512) -> ("Array Out"=w503:i8[][])  [unwired: 1 in, 1 out]
                n176 = Get Queue Status(queue=w486, error in (no error)=w487) -> (queue out=w485:refnum<queue>, # elements in queue=w484:i32)  [unwired: 1 in, 6 out]
                n177 = Compound Arithmetic op=ADD(w506, w505, w504, w503) -> (w483:i8[][])
                n178 = expression code="x*2"(w483) -> (w481:i8[][])
                n179 = Multiply(x=w482, y=w481) -> (x*y=w480:i8[][])
                n180 = local write "SF queue"(w484) -> ()
                n181 = local read "stop out"() -> (w520:bool)
                n182 = Bundle(w501, w480) -> (w500:cluster{bool, i8[][]})  [unwired: 1 in]
                n183 = Lossy Enqueue Element(queue=w502, element=w500) -> ()  [unwired: 1 in, 4 out]
                "SF Index" <- w499
              }
              n184 = while {
                tunnel: [w465] -> w431
                tunnel: w433 -> [w467]
                tunnel: w429 -> [w472]
                tunnel: u16 13 ("bits A/D") -> [w463]
                i -> [w468]
                stop <- w473 stop-if-true
                # "Log compress and display data"
                n185 = Dequeue Element(queue=w467, timeout in ms (-1)=5000) -> (queue out=w466:refnum<queue>, element=w471:cluster{bool, "Array":i16[][]})  [unwired: 1 in, 2 out]
                n186 = Get Queue Status(queue=w466) -> (queue out=w465:refnum<queue>, # elements in queue=→"Display queue":i32)  [unwired: 2 in, 6 out]
                n187 = Unbundle(w471) -> (w470:bool, "Array"=w469:i16[][])
                n188 = case shown="True" w470 {
                  tunnel: [w477 w479] -> w475
                  tunnel: w469 -> [w477 w478]
                  frame False {
                  }
                  frame True {
                    n189 = call "ReverseData.vi"("Array in"=w478) -> ("Array out"=w479:i16[][])
                  }
                }
                n190 = Increment(x=w468) -> (x+1=w476:i32)
                n191 = call "CurrentPlane.vi"("bits A/D"=w463, "Axis Vals"=w472, "Frame"=w476, "Data"=w475) -> ("stop out"=w473:bool)  [unwired: 6 in, 1 out]
                n192 = local write "stop out"(w473) -> ()
                "Display index" <- w468
              }
              n193 = while {
                tunnel: w451 -> [w553]
                tunnel: w450 -> [w545]
                tunnel: w452 -> [w554]
                tunnel: w460 -> [w552]
                tunnel: ["stop out"] -> w459
                tunnel: w428 -> [w521]
                tunnel: w453 -> [w530]
                tunnel: w436 -> [w533]
                tunnel: w435 -> [w532]
                i -> [w534]
                stop <- "stop out" stop-if-true
                # "Get next available frame and queue data"
                n194 = call <instrlib>:"niScope Initiate Acquisition.vi"("instrument handle"=w533) -> ("instrument handle out"=w536:refnum<k15>, "error out"=w537:errorcluster)  [unwired: 2 in, 11 out]
                n195 = call <instrlib>:"niScope Initiate Acquisition.vi"("instrument handle"=w532, "error in"=w537) -> ("instrument handle out"=w535:refnum<k15>, "error out"=w546:errorcluster)  [unwired: 1 in, 11 out]
                n196 = call "Rapid Read_NI.vi"("Channel"="0", "lines per plane"=w553, "error in"=w546, "rf points per line"=w545, "Motion Board ID"=w554, "NI Card"=w521) -> ("error out"=w523:errorcluster, "Reverse?"=w550:bool, "Array"=w528:i8[][], "dig gain"=w548:dbl)  [unwired: 2 in]
                n197 = Bundle("dig gain"=w548, "Reverse?"=w550) -> (w549:cluster{"dig gain":dbl, "Reverse?":bool})  [unwired: 1 out]
                n198 = Lossy Enqueue Element(queue=w530, element=w528) -> (queue out=w529:refnum<queue>, error out=w527:errorcluster)  [unwired: 1 in, 2 out]
                n199 = Lossy Enqueue Element(queue=w552, element=w549, error in (no error)=w523) -> (error out=w522:errorcluster)  [unwired: 3 out]
                n200 = flat-sequence {
                  tunnel: w545 -> [w565]
                  tunnel: [w564] -> w541
                  tunnel: [w563] -> w540
                  tunnel: [w562] -> w539
                  tunnel: [w561] -> w538
                  tunnel: w536 -> [w556]
                  tunnel: w535 -> [w560]
                  tunnel: 0 -> [w559]
                  tunnel: w522 -> [_]
                  tunnel: w521 -> [w558]
                  frame #0 {
                    w555 = "1" ("Channel")
                    n201 = call-poly <instrlib>:"niScope Fetch (poly).vi"("timeout"=w559, "numSamples"=w565, "channels"="1" ("Channel"), "instrument handle"=w558) -> ("wfm"=w564:i8[][])  [unwired: 1 in, 6 out]
                    n202 = call-poly <instrlib>:"niScope Fetch (poly).vi"("timeout"=w559, "numSamples"=w565, "instrument handle"=w556) -> ("wfm"=w563:i8[][])  [unwired: 2 in, 6 out]
                    n203 = call-poly <instrlib>:"niScope Fetch (poly).vi"("timeout"=w559, "numSamples"=w565, "channels"=w555, "instrument handle"=w556) -> ("wfm"=w562:i8[][])  [unwired: 1 in, 6 out]
                    n204 = call-poly <instrlib>:"niScope Fetch (poly).vi"("timeout"=w559, "numSamples"=w565, "channels"=w555, "instrument handle"=w560) -> ("wfm"=w561:i8[][])  [unwired: 1 in, 6 out]
                  }
                }
                n205 = Lossy Enqueue Element(queue=w529, element=w541, error in (no error)=w527) -> (queue out=w544:refnum<queue>, error out=w526:errorcluster)  [unwired: 2 out]
                n206 = Lossy Enqueue Element(queue=w544, element=w540, error in (no error)=w526) -> (queue out=w543:refnum<queue>, error out=w525:errorcluster)  [unwired: 2 out]
                n207 = Lossy Enqueue Element(queue=w543, element=w539, error in (no error)=w525) -> (queue out=w542:refnum<queue>, error out=w524:errorcluster)  [unwired: 2 out]
                n208 = Lossy Enqueue Element(queue=w542, element=w538, error in (no error)=w524) -> ()  [unwired: 4 out]
                "Read Data index" <- w534
              }
              n209 = And(x=w459, y=w458) -> (x .and. y?=w430:bool)
              n210 = Release Queue(queue=w457, force destroy? (F)=w430) -> ()  [unwired: 1 in, 3 out]
              n211 = Release Queue(queue=w439, force destroy? (F)=w430) -> ()  [unwired: 1 in, 3 out]
              n212 = Release Queue(queue=w431, force destroy? (F)=w430) -> ()  [unwired: 1 in, 3 out]
            }
            frame 1 {
              # "1T/5R test case/ This works but was a bit slower than case using flip flop gate. Also cam suffer memory overflow if Byte depth too small"
              # "Arm digitizer"
              n213 = Reverse 1D Array(array=w577) -> (reversed array=w574:void[])
              n214 = for {
                tunnel: [w644] -> w578
                tunnel: w574 -> [w643] mode=indexing
                n215 = call <instrlib>:"niScope Initiate Acquisition.vi"("instrument handle"=w643) -> ("error out"=w644:errorcluster)  [unwired: 2 in, 12 out]
              }
              n216 = Array To Cluster(array=w577) -> (cluster=w581:cluster{"[0]":void, "[1]":void, "[2]":void})
              n217 = Index Array(array=w594) -> (element=w593:T11)  [unwired: 1 in]
              n218 = Index Array(array=w594, index=1) -> (element=w589:T11)
              n219 = Index Array(array=w594, index=2) -> (element=w590:T11)
              n220 = Index Array(array=w594, index=3) -> (element=w591:T11)
              n221 = Index Array(array=w594, index=4) -> (element=w592:T11)
              n222 = Unbundle(w581) -> ("[0]"=w580, "[1]"=w576, "[2]"=w575)
              n223 = Obtain Queue(max queue size (-1, unlimited)=5, element data type=cluster{"Fetch:Records Done":i32, bool} {"Fetch:Records Done"=0, TRUE}) -> (queue out=w586:refnum<queue>)  [unwired: 2 in, 3 out]
              n224 = node-c288() -> (w571:T6)  [unwired: 4 in]
              n225 = Obtain Queue(max queue size (-1, unlimited)=25, element data type=i8[][] [] ("Array")) -> (queue out=w588:refnum<queue>)  [unwired: 2 in, 3 out]
              n226 = while {
                tunnel: w586 -> [w719]
                tunnel: [w710] -> w585
                tunnel: w580 -> [w715]
                tunnel: w576 -> [w707]
                tunnel: w575 -> [w714]
                tunnel: w588 -> [w717]
                tunnel: w600 -> [w688]
                tunnel: w599 -> [w713]
                tunnel: [w691] -> w583
                tunnel: w578 -> [w709]
                tunnel: [w698] -> w566
                i -> [w700]
                stop <- w710 stop-if-true
                w703 = 483 items=["Start"=482, "Trigger"=483, "Pretrigger"=477, "Now"=481, "Read Pointer"=388] ("Fetch:Fetch Relative To")
                w690 = 1
                # "This loop reads the data once it is in the queue"
                # "Get and display data"
                n227 = Dequeue Element(queue=w719, timeout in ms (-1)=10000, error in (no error)=w709) -> (element=w718:cluster{"Fetch:Records Done":i32, bool}, error out=w701:errorcluster)  [unwired: 2 out]
                n228 = local write "Read Data index"(w700) -> ()
                n229 = Unbundle(w718) -> ("Fetch:Records Done"=w704:i32)  [unwired: 1 out]
                n230 = property class="niScope"(reference=w715, error in=w701, "Fetch Relative To"=w703, "Fetch Record Number"=w704, "Fetch Number of Records"=w713) -> (reference out=w697:refnum<k15>, error out=w702:errorcluster)
                n231 = property class="niScope"(reference=w707, "Fetch Relative To"=w703, "Fetch Record Number"=w704, "Fetch Number of Records"=w713) -> (reference out=w705:refnum<k15>)  [unwired: 1 in, 1 out]
                n232 = call-poly <instrlib>:"niScope Fetch (poly).vi"("timeout"=w690, "error in"=w702, "numSamples"=w688, "instrument handle"=w697) -> ("error out"=w699:errorcluster, "wfm"=w708:i8[][])  [unwired: 1 in, 5 out]
                n233 = Lossy Enqueue Element(queue=w717, element=w708, error in (no error)=w699) -> (queue out=w695:refnum<queue>, error out=w696:errorcluster)  [unwired: 2 out]
                n234 = call-poly <instrlib>:"niScope Fetch (poly).vi"("timeout"=w690, "numSamples"=w688, "channels"="1", "instrument handle"=w697) -> ("wfm"=w692:i8[][])  [unwired: 1 in, 6 out]
                n235 = Lossy Enqueue Element(queue=w695, element=w692, error in (no error)=w696) -> (queue out=w693:refnum<queue>, error out=w694:errorcluster)  [unwired: 2 out]
                n236 = property class="niScope"(reference=w714, "Fetch Relative To"=w703, "Fetch Record Number"=w704, "Fetch Number of Records"=w713) -> (reference out=w706:refnum<k15>)  [unwired: 1 in, 1 out]
                n237 = stacked-sequence {
                  tunnel: [w734] -> w722
                  tunnel: [w733] -> w721
                  tunnel: [w732] -> w720
                  tunnel: w688 -> [w731]
                  tunnel: w690 -> [w730]
                  tunnel: w706 -> [w729]
                  tunnel: w705 -> [w728]
                  tunnel: [w725] -> w698
                  frame #0 {
                    n238 = call-poly <instrlib>:"niScope Fetch (poly).vi"("timeout"=w730, "numSamples"=w731, "instrument handle"=w728) -> ("wfm"=w734:i8[][])  [unwired: 2 in, 6 out]
                    n239 = call-poly <instrlib>:"niScope Fetch (poly).vi"("timeout"=w730, "numSamples"=w731, "channels"="1" ("Channel"), "instrument handle"=w728) -> ("wfm"=w733:i8[][])  [unwired: 1 in, 6 out]
                    n240 = call-poly <instrlib>:"niScope Fetch (poly).vi"("timeout"=w730, "numSamples"=w731, "channels"="1" ("Channel"), "instrument handle"=w729) -> ("error out"=w725:errorcluster, "wfm"=w732:i8[][])  [unwired: 1 in, 5 out]
                  }
                }
                n241 = Lossy Enqueue Element(queue=w693, element=w722, error in (no error)=w694) -> (queue out=w724:refnum<queue>, error out=w712:errorcluster)  [unwired: 2 out]
                n242 = local read "stop out"() -> (w710:bool)
                n243 = Lossy Enqueue Element(queue=w724, element=w721, error in (no error)=w712) -> (queue out=w723:refnum<queue>, error out=w711:errorcluster)  [unwired: 2 out]
                n244 = Lossy Enqueue Element(queue=w723, element=w720, error in (no error)=w711) -> (queue out=w691:refnum<queue>)  [unwired: 3 out]
              }
              n245 = timed-loop {
                shift-right: [w617] -> _
                shift-left: 0 -> [w625]
                shift-right: [w632] -> _
                shift-left: TRUE -> [w626]
                tunnel: w603 -> [w630]
                tunnel: w586 -> [w621]
                tunnel: [w624] -> w572
                tunnel: [w611] -> w584
                tunnel: w580 -> [w623]
                tunnel: w579 -> [w618]
                tunnel: w578 -> [w628]
                timing: w571 -> [_]
                timing-out: [_] -> w570
                i -> [w610]
                stop <- w624 stop-if-true
                # "This loop performs back and forth scan and records record # at end of run"
                n246 = Bundle(w625, w626) -> (w622:cluster{i32, bool})  [unwired: 1 in]
                n247 = Select(t=T5 6 ("Program (1)"), s=w626, f=T5 7 ("Program (1)")) -> (s? t:f=w629:T5)
                n248 = call <vilib>:"Run Program.flx"("error in (no error)"=w628, "Program (1)"=w629, "Board ID"=w630) -> ("error out"=w620:errorcluster, "Bd ID Out"=w615:T2)  [unwired: 4 out]
                n249 = stacked-sequence {
                  tunnel: w620 -> [w636]
                  tunnel: [w636] -> w619
                  tunnel: [w634] -> w616
                  tunnel: w615 -> [w634]
                  frame #0 {
                    n250 = Wait (ms)(milliseconds to wait=20) -> ()  [unwired: 1 out]
                  }
                }
                n251 = call-poly <vilib>:"Wait for Move Complete.flx"("Poll Interval (20 ms)"=5, "error in (no error)"=w619, "Axis or Vector Space"=w618, "Board ID"=w616) -> ("error out"=w627:errorcluster)  [unwired: 4 in, 3 out]
                n252 = property class="niScope"(reference=w623, error in=w627) -> (error out=w614:errorcluster, "Records Done"=w617:i32)  [unwired: 1 out]
                n253 = local read "stop out"() -> (w624:bool)
                n254 = Lossy Enqueue Element(queue=w621, element=w622, error in (no error)=w614) -> (queue out=w612:refnum<queue>, error out=w609:errorcluster)  [unwired: 2 out]
                n255 = Not(x=w626) -> (.not. x?=w632:bool)
                n256 = Get Queue Status(queue=w612, error in (no error)=w609) -> (queue out=w611:refnum<queue>, # elements in queue=→"Record queue":i32)  [unwired: 1 in, 6 out]
                "Read Loop" <- w610
              }
              n257 = while {
                tunnel: w588 -> [w684]
                tunnel: [w648] -> w587
                tunnel: w592 -> [w677]
                tunnel: w591 -> [w676]
                tunnel: w593 -> [w675]
                tunnel: w589 -> [w674]
                tunnel: w590 -> [w673]
                tunnel: w578 -> [w663]
                shift-right: [w649] -> _
                shift-left: TRUE -> [w647]
                tunnel: w568 -> [w650]
                tunnel: u16 13 ("bits A/D") -> [w646]
                i -> [w652]
                stop <- w648 stop-if-true
                w658 = 100
                # "This loop does beam forming after data is read."
                n258 = Dequeue Element(queue=w684, timeout in ms (-1)=10000, error in (no error)=w663) -> (queue out=w664:refnum<queue>, element=w665:i8[][], error out=w667:errorcluster)  [unwired: 1 out]
                n259 = Dequeue Element(queue=w664, timeout in ms (-1)=w658, error in (no error)=w667) -> (queue out=w683:refnum<queue>, element=w680:i8[][], error out=w662:errorcluster)  [unwired: 1 out]
                n260 = call "TimeShiftData.vi"("output cluster"=w674, "Array In"=w680) -> ("Array Out"=w671:i16[][])  [unwired: 2 in]
                n261 = call "TimeShiftData.vi"("output cluster"=w675, "Array In"=w665) -> ("Array Out"=w672:i16[][])  [unwired: 2 in]
                n262 = Dequeue Element(queue=w683, timeout in ms (-1)=w658, error in (no error)=w662) -> (queue out=w682:refnum<queue>, element=w679:i8[][], error out=w661:errorcluster)  [unwired: 1 out]
                n263 = call "TimeShiftData.vi"("output cluster"=w673, "Array In"=w679) -> ("Array Out"=w670:i16[][])  [unwired: 2 in]
                n264 = Dequeue Element(queue=w682, timeout in ms (-1)=w658, error in (no error)=w661) -> (queue out=w681:refnum<queue>, element=w660:i8[][], error out=w659:errorcluster)  [unwired: 1 out]
                n265 = call "TimeShiftData.vi"("output cluster"=w676, "Array In"=w660) -> ("Array Out"=w669:i16[][])  [unwired: 2 in]
                n266 = Dequeue Element(queue=w681, timeout in ms (-1)=w658, error in (no error)=w659) -> (queue out=w657:refnum<queue>, element=w678:i8[][], error out=w656:errorcluster)  [unwired: 1 out]
                n267 = call "TimeShiftData.vi"("output cluster"=w677, "Array In"=w678) -> ("Array Out"=w668:i16[][])  [unwired: 2 in]
                n268 = Get Queue Status(queue=w657, error in (no error)=w656) -> (# elements in queue=→"SF queue":i32)  [unwired: 1 in, 7 out]
                n269 = Compound Arithmetic op=ADD(w672, w671, w670, w669, w668) -> (w651:i16[][])
                n270 = case shown="True" w647 {
                  tunnel: [w685 w687] -> w653
                  tunnel: w651 -> [w685 w686]
                  frame False {
                  }
                  frame True {
                    n271 = call "ReverseData.vi"("Array in"=w686) -> ("Array out"=w687:i16[][])
                  }
                }
                n272 = Increment(x=w652) -> (x+1=w654:i32)
                n273 = local write "SF Index"(w652) -> ()
                n274 = call "CurrentPlane.vi"("gain"=1.0, "bits A/D"=w646, "Axis Vals"=w650, "Frame"=w654, "Data"=w653) -> ("stop out"=w648:bool)  [unwired: 5 in, 1 out]
                n275 = local write "stop out"(w648) -> ()
                n276 = Not(x=w647) -> (.not. x?=w649:bool)
              }
              n277 = node-c288(w570) -> ()
              n278 = Compound Arithmetic op=AND(w572, w585, w587) -> (w573:bool)
              n279 = Release Queue(queue=w584, force destroy? (F)=w573) -> ()  [unwired: 1 in, 3 out]
              n280 = for {
                tunnel: w577 -> [w642] mode=indexing
                tunnel: w566 -> [w641]
                n281 = call <instrlib>:"niScope Abort.vi"("instrument handle"=w642, "error in"=w641) -> ()  [unwired: 12 in, 2 out]
              }
              n282 = Release Queue(queue=w583, force destroy? (F)=w573) -> ()  [unwired: 1 in, 3 out]
            }
            frame 2 {
              w746 = 10
              w741 = 2 ("index")
              w770 = 5
              w748 = "0,1"
              # "Restructure file names"
              # "Read queue and send to files. About same as reading channel by channel"
              n283 = Reshape Array(w771, w770, w770) -> (w739:T12)
              n284 = expression code="x*5"(w761) -> (w772:dbl)
              n285 = Index Array(array=w739, index (col)=4 ("index")) -> (element=w745:T13)  [unwired: 1 in]
              n286 = Initialize Array(i16 0, w761, w738) -> (w759:i16[][])
              n287 = Array Subset(array=w739, index (col)=w741, length (col)=w741) -> (w744:T12)  [unwired: 2 in]
              n288 = Array Subset(array=w739, length (col)=2 ("index")) -> (w743:T12)  [unwired: 3 in]
              n289 = call "RTHeader.vi"("Comment"="Full 25") -> ("Header String Out"=w735:string)  [unwired: 5 in, 1 out]
              n290 = Obtain Queue(max queue size (-1, unlimited)=15, element data type=T9 {"gain"=0.0, "wfm"=[], TRUE, "max queue size (-1, unlimited)"=15}) -> (queue out=w776:refnum<queue>)  [unwired: 3 in, 2 out]
              n291 = New Data Value Reference(data value=w759) -> (data value reference=w758:refnum<data-value>)  [unwired: 1 in, 1 out]
              n292 = Reshape Array(w743, w746) -> (w747:T13)
              n293 = Build Array(w749, w774, w773) -> (w779:void[])
              n294 = Reshape Array(w744, w746) -> (w756:T13)
              n295 = Obtain Queue(max queue size (-1, unlimited)=5, element data type=cluster{"gain":dbl, bool, "wfm":i16[][]} {"gain"=0.0, TRUE, "wfm"=[]}) -> (queue out=w760:refnum<queue>)  [unwired: 3 in, 2 out]
              n296 = Build Array(w748, w748, "1") -> (w778:string[])
              n297 = Tick Count (ms)() -> (millisecond timer value=w753:u32)
              n298 = Build Array(w747, w756, w745) -> (w755:T12)
              n299 = while {
                tunnel: w776 -> [w798]
                tunnel: w738 -> [w797]
                tunnel: [w793] -> w765
                tunnel: w761 -> [w796]
                tunnel: w758 -> [w792]
                tunnel: w760 -> [w795]
                tunnel: w755 -> [w787]
                tunnel: i32[] [10, 10, 5] -> [w791]
                shift-right: [w789] -> _
                shift-left: w753 -> [w790]
                tunnel: [w788] -> _
                tunnel: 10000 -> [w783]
                tunnel: [w782] -> w737
                tunnel: w735 -> [w780]
                i -> [w781]
                stop <- w793 stop-if-true
                n300 = for {
                  tunnel: w797 -> [w812]
                  tunnel: w796 -> [w822]
                  tunnel: w798 -> [w825]
                  tunnel: [w821] -> w786 mode=indexing
                  tunnel: [w811] -> w794
                  tunnel: [w820] -> w784
                  tunnel: w792 -> [w819]
                  tunnel: w787 -> [_] mode=indexing
                  tunnel: w791 -> [w815]
                  tunnel: w787 -> [w817]
                  tunnel: w783 -> [w814]
                  tunnel: w781 -> [w809]
                  tunnel: w780 -> [w807]
                  n301 = Dequeue Element(queue=w825, timeout in ms (-1)=w814) -> (element=w824:T9)  [unwired: 1 in, 3 out]
                  n302 = Unbundle(w824) -> ("gain"=w811:dbl, "wfm"=w808:i8[][], w821:bool, "max queue size (-1, unlimited)"=w806:i32)
                  n303 = Index Array(array=w815, index=w806) -> (element=w813:i32)
                  n304 = Index Array(array=w817, index (row)=w806) -> (element=w816:T13)  [unwired: 1 in]
                  n305 = Multiply(x=w812, y=w813) -> (x*y=w818:i32)
                  n306 = Reshape Array(w808, w822, w818) -> (w823:i8[][])
                  n307 = for {
                    N: w813 -> [_]
                    tunnel: w816 -> [w837]
                    tunnel: [w840] -> w820
                    tunnel: w819 -> [w839]
                    shift-right: [w832] -> _
                    shift-left: w823 -> [w842]
                    tunnel: w812 -> [w831]
                    i -> [w838]
                    n308 = Index Array(array=w837, index=w838) -> (element=w836:T11)
                    n309 = Delete From Array(array=w842, length=w831, index (col)=0 ("disabled index (col)")) -> (deleted portion=w835:i8[], array with subset deleted=w832:i8[][])  [unwired: 1 in]
                    n310 = for {
                      tunnel: w835 -> [w844] mode=indexing
                      tunnel: [w843] -> w834 mode=indexing
                      n311 = call-poly <vilib>:"Mean.vi"("X"=w844) -> ("mean"=w846:dbl)  [unwired: 1 out]
                      n312 = To Word Integer(number=w846) -> (16bit integer=w845:i16)
                      n313 = Subtract(x=w844, y=w845) -> (x-y=w843:i16)
                    }
                    n314 = call-poly "TimeShiftDataPoly.vi"("output cluster"=w836, "Array In"=w834) -> ("Array Out"=w841:i16[][])  [unwired: 2 in]
                    n315 = in-place {
                      in-place-border: w841 -> [w849]
                      n316 = in-place-dvr #1(w839) -> (w847:i16[][])  [unwired: 1 out]
                      n317 = Add(x=w849, y=w847) -> (x+y=w848:i16[][])
                      n318 = in-place-dvr #1(w848) -> (w840:refnum<data-value>)  [unwired: 1 out]
                    }
                  }
                  n319 = case shown="True" "Save Raw" {
                    tunnel: w806 -> [_ w827]
                    tunnel: w809 -> [_ w829]
                    tunnel: w808 -> [_ w826]
                    tunnel: w807 -> [_ w828]
                    frame False {
                    }
                    frame True {
                      n320 = call "RawRT_Capture.vi"("Raw data"=w826, "File Name In"="Raw Name", "DigCard"=w827, "header"=w828, "Iter"=w829) -> ()  [unwired: 7 in]
                    }
                  }
                }
                n321 = local write "SF Index"(w781) -> ()
                n322 = local read "stop out"() -> (w793:bool)
                n323 = Or Array Elements(Boolean array=w786) -> (logical OR=w785:bool)
                n324 = in-place {
                  in-place-border: w795 -> [w805]
                  in-place-border: w785 -> [w804]
                  in-place-border: w794 -> [w803]
                  n325 = in-place-dvr #2(w784) -> (w799:i16[][])  [unwired: 1 out]
                  n326 = Bundle("gain"=w803, w804, w799) -> (w802:cluster{"gain":dbl, bool, i16[][]})  [unwired: 1 in]
                  n327 = Multiply(x=i16 0, y=w799) -> (x*y=w801:i16[][])
                  n328 = Enqueue Element(queue=w805, element=w802) -> ()  [unwired: 2 in, 3 out]
                  n329 = in-place-dvr #2(w801) -> (w782:refnum<data-value>)  [unwired: 1 out]
                }
                n330 = Tick Count (ms)() -> (millisecond timer value=w789:u32)
                n331 = Subtract(x=w789, y=w790) -> (x-y=w788:u32)
              }
              n332 = while {
                tunnel: w763 -> [w917]
                tunnel: w760 -> [w911]
                tunnel: [w914] -> _
                tunnel: [w916] -> w764
                i -> [w918]
                stop <- w914 stop-if-true
                # "Slightly faster version to read data"
                # "Get and display data"
                n333 = Dequeue Element(queue=w911, timeout in ms (-1)=5000) -> (queue out=w916:refnum<queue>, element=w913:cluster{"gain":dbl, bool, "wfm":i16[][]})  [unwired: 1 in, 2 out]
                n334 = Unbundle(w913) -> ("gain"=w908:dbl, w909:bool, "wfm"=w910:i16[][])
                n335 = case shown="True" w909 {
                  tunnel: w910 -> [w919 w921]
                  tunnel: [w919 w920] -> w912
                  frame False {
                  }
                  frame True {
                    n336 = call "ReverseData.vi"("Array in"=w921) -> ("Array out"=w920:i16[][])
                  }
                }
                n337 = Increment(x=w918) -> (x+1=w907:i32)
                n338 = local write "Display index"(w907) -> ()
                n339 = call "CurrentPlane.vi"("gain"=w908, "bits A/D"=13, "Axis Vals"=w917, "Frame"=w907, "Data"=w912) -> ("stop out"=w914:bool)  [unwired: 5 in, 1 out]
                n340 = local write "stop out"(w914) -> ()
              }
              n341 = global read "MotionGlobals.vi" "DigTimeOut"() -> (w752)
              n342 = while {
                tunnel: w779 -> [w863]
                tunnel: w778 -> [w862]
                tunnel: w776 -> [w861]
                tunnel: w774 -> [w860]
                tunnel: w773 -> [w859]
                tunnel: w772 -> [w858]
                tunnel: w738 -> [w857]
                tunnel: [w856] -> w766
                tunnel: w757 -> [w854]
                shift-right: [w852] -> _
                shift-left: w753 -> [w853]
                tunnel: [w851] -> _
                tunnel: w752 -> [w850]
                stop <- w855 stop-if-true
                n343 = for {
                  tunnel: w857 -> [w876]
                  tunnel: w858 -> [w879]
                  tunnel: w863 -> [w878] mode=indexing
                  tunnel: w862 -> [w877] mode=indexing
                  tunnel: w861 -> [w875]
                  tunnel: [w871] -> _
                  tunnel: w860 -> [w870]
                  tunnel: w859 -> [w869]
                  tunnel: [w867] -> w856
                  tunnel: w854 -> [w866]
                  tunnel: w850 -> [w865]
                  i -> [w864]
                  # "Read data"
                  n344 = case shown="1, Default" w864 {
                    tunnel: w879 -> [w883 w902]
                    tunnel: w878 -> [w884 w901]
                    tunnel: w877 -> [w881 w899]
                    tunnel: w876 -> [w885 w898]
                    tunnel: [w886 w897] -> w874
                    tunnel: [w888 w896] -> w873
                    tunnel: [w887 w895] -> w871
                    tunnel: w870 -> [w892 _]
                    tunnel: w869 -> [w891 _]
                    tunnel: [w882 _] -> w868
                    tunnel: w866 -> [w880 _]
                    tunnel: w865 -> [_ w893]
                    frame 0 {
                      # "Read files and queue it up."
                      n345 = call <instrlib>:"niScope Initiate Acquisition.vi"("instrument handle"=w892) -> ("error out"=w890:errorcluster)  [unwired: 2 in, 12 out]
                      n346 = call <instrlib>:"niScope Initiate Acquisition.vi"("instrument handle"=w891, "error in"=w890) -> ("error out"=w889:errorcluster)  [unwired: 1 in, 12 out]
                      n347 = call "Rapid Read_NI.vi"("Channel"=w881, "lines per plane"=w883, "error in"=w889, "rf points per line"=w885, "Motion Board ID"=w880, "NI Card"=w884) -> ("error out"=w887:errorcluster, "Reverse?"=w882:bool, "Array"=w888:i8[][], "dig gain"=w886:dbl)  [unwired: 2 in]
                    }
                    frame 1, Default {
                      n348 = property class="niScope"(reference=w901, "Fetch Record Number"=0, "Fetch Number of Records"=w902) -> (reference out=w900:refnum<k15>, error out=w894:errorcluster)  [unwired: 1 in]
                      n349 = call-poly <instrlib>:"niScope Fetch (poly).vi"("timeout"=w893, "error in"=w894, "numSamples"=w898, "channels"=w899, "instrument handle"=w900) -> ("error out"=w895:errorcluster, "wfm"=w896:i8[][], "wfm info"=w905:T14)  [unwired: 4 out]
                      n350 = Index Array(array=w905) -> (element=w904:T15)  [unwired: 1 in]
                      n351 = Unbundle By Name(w904) -> ("gain"=w897:dbl)
                    }
                  }
                  n352 = local write "Read Data index"(w864) -> ()
                  n353 = Bundle("gain"=w874, "wfm"=w873, "Reverse?"=w868, w864) -> (w872:T16)  [unwired: 1 in]
                  n354 = Enqueue Element(queue=w875, element=w872) -> (queue out=w867:refnum<queue>)  [unwired: 2 in, 2 out]
                }
                n355 = local read "stop out"() -> (w855:bool)
                n356 = Tick Count (ms)() -> (millisecond timer value=w852:u32)
                n357 = Subtract(x=w852, y=w853) -> (x-y=w851:u32)
              }
              n358 = Release Queue(queue=w766, force destroy? (F)=w765) -> ()  [unwired: 1 in, 3 out]
              n359 = Delete Data Value Reference(data value reference=w737) -> ()  [unwired: 1 in, 2 out]
              n360 = Release Queue(queue=w764, force destroy? (F)=w765) -> ()  [unwired: 1 in, 3 out]
            }
            frame 3 {
              w932 = 2 ("index")
              w957 = 5
              # "Reduced data case that drop ring 5 receive"
              # "Restructure file names"
              # "Read queue and send to files. About same as reading channel by channel"
              n361 = Reshape Array(w958, w957, w957) -> (w930:T12)
              n362 = Initialize Array(i16 0, w927, w929) -> (w947:i16[][])
              n363 = Array Subset(array=w930, index (col)=w932, length (col)=w932) -> (w931:T12)  [unwired: 2 in]
              n364 = Array Subset(array=w930, length (col)=2 ("index")) -> (w934:T12)  [unwired: 3 in]
              n365 = Obtain Queue(max queue size (-1, unlimited)=6, element data type=T9 {"gain"=0.0, "wfm"=[], TRUE, "max queue size (-1, unlimited)"=15}) -> (queue out=w960:refnum<queue>)  [unwired: 3 in, 2 out]
              n366 = Build Array(w926, w924) -> (w925:void[])
              n367 = New Data Value Reference(data value=w947) -> (data value reference=w946:refnum<data-value>)  [unwired: 1 in, 1 out]
              n368 = Reshape Array(w934, 10) -> (w933:T13)
              n369 = Reshape Array(w931, 10) -> (w944:T13)
              n370 = Obtain Queue(max queue size (-1, unlimited)=3, element data type=cluster{"gain":dbl, bool, "wfm":i16[][]} {"gain"=0.0, TRUE, "wfm"=[]}) -> (queue out=w948:refnum<queue>)  [unwired: 3 in, 2 out]
              n371 = expression code="x*5"(w927) -> (w922:dbl)
              n372 = Tick Count (ms)() -> (millisecond timer value=w941:u32)
              n373 = Build Array(w933, w944) -> (w943:T12)
              n374 = while {
                tunnel: w960 -> [w980]
                tunnel: w929 -> [w979]
                tunnel: [w975] -> w952
                tunnel: w927 -> [w978]
                tunnel: w946 -> [w973]
                tunnel: w948 -> [w977]
                tunnel: w943 -> [w968]
                tunnel: i32[] [10, 10] -> [w972]
                shift-right: [w970] -> _
                shift-left: w941 -> [w971]
                tunnel: [w969] -> _
                tunnel: 10000 -> [w964]
                tunnel: i16[] [1, 1, 1, 1, 1, 1, 1, 1, 2, 2] -> [w963]
                tunnel: [w962] -> w928
                i -> [w974]
                stop <- w975 stop-if-true
                n375 = for {
                  tunnel: w979 -> [w991]
                  tunnel: w978 -> [w1002]
                  tunnel: w980 -> [w1005]
                  tunnel: [w1001] -> w967 mode=indexing
                  tunnel: [w1000] -> w976
                  tunnel: [w999] -> w965
                  tunnel: w973 -> [w998]
                  tunnel: w968 -> [_] mode=indexing
                  tunnel: w972 -> [w995]
                  tunnel: w968 -> [w997]
                  tunnel: w964 -> [w994]
                  tunnel: w963 -> [w990]
                  n376 = Dequeue Element(queue=w1005, timeout in ms (-1)=w994) -> (element=w1004:T9)  [unwired: 1 in, 3 out]
                  n377 = Unbundle(w1004) -> ("gain"=w1000:dbl, "wfm"=w1003:i8[][], w1001:bool, "max queue size (-1, unlimited)"=w992:i32)
                  n378 = Index Array(array=w995, index=w992) -> (element=w993:i32)
                  n379 = Index Array(array=w997, index (row)=w992) -> (element=w996:T13)  [unwired: 1 in]
                  n380 = Multiply(x=w991, y=w993) -> (x*y=w989:i32)
                  n381 = Reshape Array(w1003, w1002, w989) -> (w988:i8[][])
                  n382 = for {
                    N: w993 -> [_]
                    tunnel: w996 -> [w1013]
                    tunnel: [w1016] -> w999
                    tunnel: w998 -> [w1015]
                    shift-right: [w1006] -> _
                    shift-left: w988 -> [w1018]
                    tunnel: w990 -> [w1008] mode=indexing
                    tunnel: w991 -> [w1007]
                    i -> [w1014]
                    n383 = Index Array(array=w1013, index=w1014) -> (element=w1012:T11)
                    n384 = Delete From Array(array=w1018, length=w1007, index (col)=0 ("disabled index (col)")) -> (deleted portion=w1011:i8[], array with subset deleted=w1006:i8[][])  [unwired: 1 in]
                    n385 = for {
                      tunnel: w1011 -> [w1021] mode=indexing
                      tunnel: [w1020] -> w1010 mode=indexing
                      n386 = call-poly <vilib>:"Mean.vi"("X"=w1021) -> ("mean"=w1022:dbl)  [unwired: 1 out]
                      n387 = To Word Integer(number=w1022) -> (16bit integer=w1019:i16)
                      n388 = Subtract(x=w1021, y=w1019) -> (x-y=w1020:i16)
                    }
                    n389 = call-poly "TimeShiftDataPoly.vi"("output cluster"=w1012, "Array In"=w1010) -> ("Array Out"=w1017:i16[][])  [unwired: 2 in]
                    n390 = in-place {
                      in-place-border: w1017 -> [w1024]
                      in-place-border: w1008 -> [w1025]
                      n391 = in-place-dvr #3(w1015) -> (w1026:i16[][])  [unwired: 1 out]
                      n392 = case shown="2" w1025 {
                        selector: w1025 -> [_ w1029]
                        tunnel: w1024 -> [w1028 w1031]
                        tunnel: [w1028 w1030] -> w1023
                        frame 0, Default {
                        }
                        frame 2 {
                          n393 = Multiply(x=w1029, y=w1031) -> (x*y=w1030:i16[][])
                        }
                      }
                      n394 = Add(x=w1023, y=w1026) -> (x+y=w1027:i16[][])
                      n395 = in-place-dvr #3(w1027) -> (w1016:refnum<data-value>)  [unwired: 1 out]
                    }
                  }
                }
                n396 = local write "SF Index"(w974) -> ()
                n397 = local read "stop out"() -> (w975:bool)
                n398 = Or Array Elements(Boolean array=w967) -> (logical OR=w966:bool)
                n399 = in-place {
                  in-place-border: w977 -> [w987]
                  in-place-border: w966 -> [w986]
                  in-place-border: w976 -> [w985]
                  n400 = in-place-dvr #4(w965) -> (w981:i16[][])  [unwired: 1 out]
                  n401 = Bundle("gain"=w985, w986, w981) -> (w984:cluster{"gain":dbl, bool, i16[][]})  [unwired: 1 in]
                  n402 = Multiply(x=i16 0, y=w981) -> (x*y=w983:i16[][])
                  n403 = Enqueue Element(queue=w987, element=w984) -> ()  [unwired: 2 in, 3 out]
                  n404 = in-place-dvr #4(w983) -> (w962:refnum<data-value>)  [unwired: 1 out]
                }
                n405 = Tick Count (ms)() -> (millisecond timer value=w970:u32)
                n406 = Subtract(x=w970, y=w971) -> (x-y=w969:u32)
              }
              n407 = while {
                tunnel: w950 -> [w1095]
                tunnel: w948 -> [w1089]
                tunnel: [w1092] -> _
                tunnel: [w1094] -> w951
                i -> [w1096]
                stop <- w1092 stop-if-true
                # "Slightly faster version to read data"
                # "Get and display data"
                n408 = Dequeue Element(queue=w1089, timeout in ms (-1)=5000) -> (queue out=w1094:refnum<queue>, element=w1091:cluster{"gain":dbl, bool, "wfm":i16[][]})  [unwired: 1 in, 2 out]
                n409 = Unbundle(w1091) -> ("gain"=w1086:dbl, w1087:bool, "wfm"=w1088:i16[][])
                n410 = case shown="False" w1087 {
                  tunnel: w1088 -> [w1097 w1099]
                  tunnel: [w1097 w1098] -> w1090
                  frame False {
                  }
                  frame True {
                    n411 = call "ReverseData.vi"("Array in"=w1099) -> ("Array out"=w1098:i16[][])
                  }
                }
                n412 = Increment(x=w1096) -> (x+1=w1085:i32)
                n413 = local write "Display index"(w1085) -> ()
                n414 = call "CurrentPlane.vi"("gain"=w1086, "bits A/D"=13, "Axis Vals"=w1095, "Frame"=w1085, "Data"=w1090) -> ("stop out"=w1092:bool)  [unwired: 5 in, 1 out]
                n415 = local write "stop out"(w1092) -> ()
              }
              n416 = global read "MotionGlobals.vi" "DigTimeOut"() -> (w940)
              n417 = while {
                tunnel: w925 -> [w1044]
                tunnel: w960 -> [w1043]
                tunnel: w924 -> [w1042]
                tunnel: w929 -> [w1041]
                tunnel: [w1040] -> w953
                tunnel: w945 -> [w1038]
                shift-right: [w1036] -> _
                shift-left: w941 -> [w1037]
                tunnel: [w1035] -> _
                tunnel: w940 -> [w1034]
                tunnel: "0,1" -> [w1033]
                tunnel: w922 -> [w1032]
                stop <- w1039 stop-if-true
                n418 = for {
                  tunnel: w1041 -> [w1057]
                  tunnel: w1044 -> [w1059] mode=indexing
                  tunnel: w1033 -> [w1058]
                  tunnel: w1043 -> [w1056]
                  tunnel: [w1052] -> _
                  tunnel: w1042 -> [w1051]
                  tunnel: [w1049] -> w1040
                  tunnel: w1038 -> [w1048]
                  tunnel: w1034 -> [w1047]
                  tunnel: w1032 -> [w1045]
                  i -> [w1046]
                  # "Read data"
                  n419 = case shown="1, Default" w1046 {
                    tunnel: w1059 -> [w1066 w1075]
                    tunnel: w1058 -> [w1064 w1074]
                    tunnel: w1057 -> [w1067 w1080]
                    tunnel: [w1068 w1079] -> w1055
                    tunnel: [w1061 w1073] -> w1054
                    tunnel: [w1069 w1078] -> w1052
                    tunnel: w1051 -> [w1070 _]
                    tunnel: [w1065 _] -> w1050
                    tunnel: w1048 -> [w1063 _]
                    tunnel: w1047 -> [_ w1076]
                    tunnel: w1045 -> [w1060 w1071]
                    frame 0 {
                      # "Read files and queue it up."
                      n420 = call <instrlib>:"niScope Initiate Acquisition.vi"("instrument handle"=w1070) -> ("error out"=w1062:errorcluster)  [unwired: 2 in, 12 out]
                      n421 = call "Rapid Read_NI.vi"("Channel"=w1064, "lines per plane"=w1060, "error in"=w1062, "rf points per line"=w1067, "Motion Board ID"=w1063, "NI Card"=w1066) -> ("error out"=w1069:errorcluster, "Reverse?"=w1065:bool, "Array"=w1061:i8[][], "dig gain"=w1068:dbl)  [unwired: 2 in]
                    }
                    frame 1, Default {
                      n422 = property class="niScope"(reference=w1075, "Fetch Record Number"=0, "Fetch Number of Records"=w1071) -> (reference out=w1081:refnum<k15>, error out=w1077:errorcluster)  [unwired: 1 in]
                      n423 = call-poly <instrlib>:"niScope Fetch (poly).vi"("timeout"=w1076, "error in"=w1077, "numSamples"=w1080, "channels"=w1074, "instrument handle"=w1081) -> ("error out"=w1078:errorcluster, "wfm"=w1073:i8[][], "wfm info"=w1083:T14)  [unwired: 4 out]
                      n424 = Index Array(array=w1083) -> (element=w1082:T15)  [unwired: 1 in]
                      n425 = Unbundle By Name(w1082) -> ("gain"=w1079:dbl)
                    }
                  }
                  n426 = local write "Read Data index"(w1046) -> ()
                  n427 = Bundle("gain"=w1055, "wfm"=w1054, "Reverse?"=w1050, w1046) -> (w1053:T16)  [unwired: 1 in]
                  n428 = Enqueue Element(queue=w1056, element=w1053) -> (queue out=w1049:refnum<queue>)  [unwired: 2 in, 2 out]
                }
                n429 = local read "stop out"() -> (w1039:bool)
                n430 = Tick Count (ms)() -> (millisecond timer value=w1036:u32)
                n431 = Subtract(x=w1036, y=w1037) -> (x-y=w1035:u32)
              }
              n432 = Release Queue(queue=w953, force destroy? (F)=w952) -> ()  [unwired: 1 in, 3 out]
              n433 = Release Queue(queue=w951, force destroy? (F)=w952) -> ()  [unwired: 1 in, 3 out]
              n434 = Delete Data Value Reference(data value reference=w928) -> ()  [unwired: 1 in, 2 out]
            }
            frame 4 {
              w1127 = 5
              # "Reduced data case that drop ring3,4,5 receive"
              # "Restructure file names"
              # "Read queue and send to files. About same as reading channel by channel"
              n435 = Reshape Array(w1128, w1127, w1127) -> (w1102:T12)
              n436 = expression code="x*5"(w1111) -> (w1105:dbl)
              n437 = Initialize Array(i16 0, w1111, w1101) -> (w1117:i16[][])
              n438 = Array Subset(array=w1102, length (col)=2 ("index")) -> (w1107:T12)  [unwired: 3 in]
              n439 = Obtain Queue(max queue size (-1, unlimited)=5, element data type=cluster{"gain":dbl, "wfm":i8[][], bool} {"gain"=0.0, "wfm"=[], TRUE}) -> (queue out=w1130:refnum<queue>)  [unwired: 3 in, 2 out]
              n440 = New Data Value Reference(data value=w1117) -> (data value reference=w1116:refnum<data-value>)  [unwired: 1 in, 1 out]
              n441 = Obtain Queue(max queue size (-1, unlimited)=5, element data type=cluster{"gain":dbl, bool, "wfm":i16[][]} {"gain"=0.0, TRUE, "wfm"=[]}) -> (queue out=w1118:refnum<queue>)  [unwired: 3 in, 2 out]
              n442 = Tick Count (ms)() -> (millisecond timer value=w1114:u32)
              n443 = Reshape Array(w1107, 10) -> (w1103:T13)
              n444 = while {
                tunnel: w1106 -> [w1202]
                tunnel: w1130 -> [w1201]
                tunnel: w1105 -> [w1200]
                tunnel: w1101 -> [w1199]
                tunnel: [w1198] -> w1123
                tunnel: w1115 -> [w1196]
                shift-right: [w1194] -> _
                shift-left: w1114 -> [w1195]
                tunnel: [w1193] -> _
                tunnel: "0,1" -> [w1192]
                i -> [w1187]
                stop <- w1197 stop-if-true
                # "Read files and queue it up."
                # "Read data"
                n445 = local write "Read Data index"(w1187) -> ()
                n446 = call "Rapid Read_NI.vi"("Channel"=w1192, "lines per plane"=w1200, "rf points per line"=w1199, "Motion Board ID"=w1196, "NI Card"=w1202) -> ("Reverse?"=w1188:bool, "Array"=w1190:i8[][], "dig gain"=w1191:dbl)  [unwired: 3 in, 1 out]
                n447 = local read "stop out"() -> (w1197:bool)
                n448 = Bundle("dig gain"=w1191, "Array"=w1190, "Reverse?"=w1188) -> (w1189:T17)  [unwired: 1 in]
                n449 = Tick Count (ms)() -> (millisecond timer value=w1194:u32)
                n450 = Enqueue Element(queue=w1201, element=w1189) -> (queue out=w1198:refnum<queue>)  [unwired: 2 in, 2 out]
                n451 = Subtract(x=w1194, y=w1195) -> (x-y=w1193:u32)
              }
              n452 = while {
                tunnel: w1130 -> [w1153]
                tunnel: w1101 -> [w1152]
                tunnel: [w1148] -> w1122
                tunnel: w1111 -> [w1151]
                tunnel: w1116 -> [w1146]
                tunnel: w1118 -> [w1150]
                tunnel: w1103 -> [w1133]
                shift-right: [w1144] -> _
                shift-left: w1114 -> [w1145]
                tunnel: [w1143] -> _
                tunnel: 10000 -> [w1141]
                tunnel: i16[] [1, 1, 1, 1, 2, 2, 2, 2, 2, 2] -> [w1140]
                tunnel: 10 -> [w1134]
                tunnel: [w1132] -> w1100
                i -> [w1147]
                stop <- w1148 stop-if-true
                n453 = Dequeue Element(queue=w1153, timeout in ms (-1)=w1141) -> (element=w1139:cluster{"gain":dbl, "wfm":i8[][], bool})  [unwired: 1 in, 3 out]
                n454 = local write "SF Index"(w1147) -> ()
                n455 = Unbundle(w1139) -> ("gain"=w1149:dbl, "wfm"=w1138:i8[][], w1135:bool)
                n456 = Multiply(x=w1152, y=w1134) -> (x*y=w1136:i32)
                n457 = Reshape Array(w1138, w1151, w1136) -> (w1137:i8[][])
                n458 = for {
                  N: w1134 -> [_]
                  tunnel: w1133 -> [w1161]
                  tunnel: [w1164] -> w1142
                  tunnel: w1146 -> [w1163]
                  shift-right: [w1156] -> _
                  shift-left: w1137 -> [w1166]
                  tunnel: w1152 -> [w1155]
                  tunnel: w1140 -> [w1154] mode=indexing
                  i -> [w1162]
                  n459 = Index Array(array=w1161, index=w1162) -> (element=w1160:T11)
                  n460 = Delete From Array(array=w1166, length=w1155, index (col)=0 ("disabled index (col)")) -> (deleted portion=w1159:i8[], array with subset deleted=w1156:i8[][])  [unwired: 1 in]
                  n461 = for {
                    tunnel: w1159 -> [w1169] mode=indexing
                    tunnel: [w1168] -> w1158 mode=indexing
                    n462 = call-poly <vilib>:"Mean.vi"("X"=w1169) -> ("mean"=w1170:dbl)  [unwired: 1 out]
                    n463 = To Word Integer(number=w1170) -> (16bit integer=w1167:i16)
                    n464 = Subtract(x=w1169, y=w1167) -> (x-y=w1168:i16)
                  }
                  n465 = call-poly "TimeShiftDataPoly.vi"("output cluster"=w1160, "Array In"=w1158) -> ("Array Out"=w1165:i16[][])  [unwired: 2 in]
                  n466 = in-place {
                    in-place-border: w1165 -> [w1172]
                    in-place-border: w1154 -> [w1173]
                    n467 = in-place-dvr #5(w1163) -> (w1174:i16[][])  [unwired: 1 out]
                    n468 = case shown="2" w1173 {
                      selector: w1173 -> [_ w1177]
                      tunnel: w1172 -> [w1176 w1179]
                      tunnel: [w1176 w1178] -> w1171
                      frame 0, Default {
                      }
                      frame 2 {
                        n469 = Multiply(x=w1177, y=w1179) -> (x*y=w1178:i16[][])
                      }
                    }
                    n470 = Add(x=w1171, y=w1174) -> (x+y=w1175:i16[][])
                    n471 = in-place-dvr #5(w1175) -> (w1164:refnum<data-value>)  [unwired: 1 out]
                  }
                }
                n472 = local read "stop out"() -> (w1148:bool)
                n473 = in-place {
                  in-place-border: w1150 -> [w1186]
                  in-place-border: w1135 -> [w1185]
                  in-place-border: w1149 -> [w1184]
                  n474 = in-place-dvr #6(w1142) -> (w1180:i16[][])  [unwired: 1 out]
                  n475 = Bundle("gain"=w1184, w1185, w1180) -> (w1183:cluster{"gain":dbl, bool, i16[][]})  [unwired: 1 in]
                  n476 = Multiply(x=i16 0, y=w1180) -> (x*y=w1182:i16[][])
                  n477 = Enqueue Element(queue=w1186, element=w1183) -> ()  [unwired: 2 in, 3 out]
                  n478 = in-place-dvr #6(w1182) -> (w1132:refnum<data-value>)  [unwired: 1 out]
                }
                n479 = Tick Count (ms)() -> (millisecond timer value=w1144:u32)
                n480 = Subtract(x=w1144, y=w1145) -> (x-y=w1143:u32)
              }
              n481 = while {
                tunnel: w1120 -> [w1214]
                tunnel: w1118 -> [w1208]
                tunnel: [w1211] -> _
                tunnel: [w1213] -> w1121
                i -> [w1215]
                stop <- w1211 stop-if-true
                # "Slightly faster version to read data"
                # "Get and display data"
                n482 = Dequeue Element(queue=w1208, timeout in ms (-1)=5000) -> (queue out=w1213:refnum<queue>, element=w1210:cluster{"gain":dbl, bool, "wfm":i16[][]})  [unwired: 1 in, 2 out]
                n483 = Unbundle(w1210) -> ("gain"=w1205:dbl, w1206:bool, "wfm"=w1207:i16[][])
                n484 = case shown="False" w1206 {
                  tunnel: w1207 -> [w1216 w1218]
                  tunnel: [w1216 w1217] -> w1209
                  frame False {
                  }
                  frame True {
                    n485 = call "ReverseData.vi"("Array in"=w1218) -> ("Array out"=w1217:i16[][])
                  }
                }
                n486 = Increment(x=w1215) -> (x+1=w1204:i32)
                n487 = local write "Display index"(w1204) -> ()
                n488 = call "CurrentPlane.vi"("gain"=w1205, "bits A/D"=13, "Axis Vals"=w1214, "Frame"=w1204, "Data"=w1209) -> ("stop out"=w1211:bool)  [unwired: 5 in, 1 out]
                n489 = local write "stop out"(w1211) -> ()
              }
              n490 = Release Queue(queue=w1123, force destroy? (F)=w1122) -> ()  [unwired: 1 in, 3 out]
              n491 = Release Queue(queue=w1121, force destroy? (F)=w1122) -> ()  [unwired: 1 in, 3 out]
              n492 = Delete Data Value Reference(data value reference=w1100) -> ()  [unwired: 1 in, 2 out]
            }
            frame 5 {
              w1239 = 5
              w1223 = "1"
              # "Read queue and send to files."
              n493 = expression code="x*5"(w1229) -> (w1241:dbl)
              n494 = Reshape Array(w1240, w1239, w1239) -> (w1238:T12)
              n495 = Initialize Array(i16 0, w1229, w1221) -> (w1227:i16[][])
              n496 = Obtain Queue(max queue size (-1, unlimited)=25, element data type=T9 {"gain"=0.0, "wfm"=[], TRUE, "max queue size (-1, unlimited)"=25}) -> (queue out=w1247:refnum<queue>)  [unwired: 3 in, 2 out]
              n497 = New Data Value Reference(data value=w1227) -> (data value reference=w1226:refnum<data-value>)  [unwired: 1 in, 1 out]
              n498 = Build Array(w1222, w1222, w1243, w1243, w1242) -> (w1250:void[])
              n499 = expression code="x*5"(w1221) -> (w1245:dbl)
              n500 = Obtain Queue(max queue size (-1, unlimited)=5, element data type=cluster{"gain":dbl, bool, "wfm":i16[][]} {"gain"=0.0, TRUE, "wfm"=[]}) -> (queue out=w1228:refnum<queue>)  [unwired: 3 in, 2 out]
              n501 = Tick Count (ms)() -> (millisecond timer value=w1224:u32)
              n502 = Build Array("0", w1223, "0", w1223, w1223) -> (w1249:string[])
              n503 = while {
                tunnel: w1250 -> [w1319]
                tunnel: w1249 -> [w1318]
                tunnel: w1247 -> [w1317]
                tunnel: w1243 -> [w1316]
                tunnel: w1242 -> [w1315]
                tunnel: w1241 -> [w1314]
                tunnel: w1221 -> [w1313]
                tunnel: [w1312] -> w1234
                tunnel: w1225 -> [w1310]
                shift-right: [w1308] -> _
                shift-left: w1224 -> [w1309]
                tunnel: [w1307] -> _
                stop <- w1311 stop-if-true
                n504 = for {
                  tunnel: w1313 -> [w1331]
                  tunnel: w1314 -> [w1334]
                  tunnel: w1319 -> [w1333] mode=indexing
                  tunnel: w1318 -> [w1332] mode=indexing
                  tunnel: w1317 -> [w1330]
                  tunnel: [w1326] -> _
                  tunnel: w1316 -> [w1325]
                  tunnel: w1315 -> [w1324]
                  tunnel: [w1322] -> w1312
                  tunnel: w1310 -> [w1321]
                  i -> [w1320]
                  # "Read data"
                  n505 = case shown="0" w1320 {
                    tunnel: w1334 -> [w1338 w1357]
                    tunnel: w1333 -> [w1339 w1356]
                    tunnel: w1332 -> [w1336 w1354]
                    tunnel: w1331 -> [w1340 w1353]
                    tunnel: [w1341 w1352] -> w1329
                    tunnel: [w1343 w1351] -> w1328
                    tunnel: [w1342 w1350] -> w1326
                    tunnel: w1325 -> [w1347 _]
                    tunnel: w1324 -> [w1346 _]
                    tunnel: [w1337 _] -> w1323
                    tunnel: w1321 -> [w1335 _]
                    frame 0 {
                      # "Read files and queue it up."
                      n506 = call <instrlib>:"niScope Initiate Acquisition.vi"("instrument handle"=w1347) -> ("error out"=w1345:errorcluster)  [unwired: 2 in, 12 out]
                      n507 = call <instrlib>:"niScope Initiate Acquisition.vi"("instrument handle"=w1346, "error in"=w1345) -> ("error out"=w1344:errorcluster)  [unwired: 1 in, 12 out]
                      n508 = call "Rapid Read_NI.vi"("Channel"=w1336, "lines per plane"=w1338, "error in"=w1344, "rf points per line"=w1340, "Motion Board ID"=w1335, "NI Card"=w1339) -> ("error out"=w1342:errorcluster, "Reverse?"=w1337:bool, "Array"=w1343:i8[][], "dig gain"=w1341:dbl)  [unwired: 2 in]
                    }
                    frame 1, Default {
                      n509 = property class="niScope"(reference=w1356, "Fetch Record Number"=0, "Fetch Number of Records"=w1357) -> (reference out=w1355:refnum<k15>, error out=w1349:errorcluster)  [unwired: 1 in]
                      n510 = call-poly <instrlib>:"niScope Fetch (poly).vi"("timeout"=0.0, "error in"=w1349, "numSamples"=w1353, "channels"=w1354, "instrument handle"=w1355) -> ("error out"=w1350:errorcluster, "wfm"=w1351:i8[][], "wfm info"=w1360:T14)  [unwired: 4 out]
                      n511 = Index Array(array=w1360) -> (element=w1359:T15)  [unwired: 1 in]
                      n512 = Unbundle By Name(w1359) -> ("gain"=w1352:dbl)
                    }
                  }
                  n513 = local write "Read Data index"(w1320) -> ()
                  n514 = Bundle("gain"=w1329, "wfm"=w1328, "Reverse?"=w1323, w1320) -> (w1327:T16)  [unwired: 1 in]
                  n515 = Enqueue Element(queue=w1330, element=w1327) -> (queue out=w1322:refnum<queue>)  [unwired: 2 in, 2 out]
                }
                n516 = local read "stop out"() -> (w1311:bool)
                n517 = Tick Count (ms)() -> (millisecond timer value=w1308:u32)
                n518 = Subtract(x=w1308, y=w1309) -> (x-y=w1307:u32)
              }
              n519 = while {
                tunnel: w1247 -> [w1267]
                tunnel: w1245 -> [w1266]
                tunnel: w1238 -> [w1254]
                tunnel: [w1262] -> w1233
                tunnel: w1229 -> [w1265]
                tunnel: w1226 -> [w1260]
                tunnel: w1228 -> [w1264]
                shift-right: [w1257] -> _
                shift-left: w1224 -> [w1258]
                tunnel: [w1256] -> _
                tunnel: w1221 -> [w1255]
                tunnel: [w1251] -> w1220
                i -> [w1261]
                stop <- w1262 stop-if-true
                n520 = for {
                  tunnel: w1266 -> [w1289]
                  tunnel: w1265 -> [w1283]
                  tunnel: w1267 -> [w1288]
                  tunnel: w1254 -> [_] mode=indexing
                  tunnel: [w1282] -> w1252 mode=indexing
                  tunnel: [w1281] -> w1263
                  tunnel: [w1280] -> w1259
                  tunnel: w1260 -> [w1279]
                  tunnel: w1255 -> [w1278]
                  tunnel: w1254 -> [w1277]
                  workers-P: _ -> [_]
                  n521 = Dequeue Element(queue=w1288, timeout in ms (-1)=10000) -> (element=w1287:T9)  [unwired: 1 in, 3 out]
                  n522 = Unbundle(w1287) -> ("gain"=w1281:dbl, "wfm"=w1286:i8[][], w1282:bool, "max queue size (-1, unlimited)"=w1275:i32)
                  n523 = Index Array(array=w1277, index (row)=w1275) -> (element=w1276:T13)  [unwired: 1 in]
                  n524 = Reshape Array(w1286, w1283, w1289) -> (w1285:i8[][])
                  n525 = for {
                    tunnel: w1276 -> [w1298] mode=indexing
                    tunnel: [w1296] -> w1280
                    tunnel: w1279 -> [w1295]
                    tunnel: w1278 -> [w1291]
                    shift-right: [w1290] -> _
                    shift-left: w1285 -> [w1299]
                    n526 = Delete From Array(array=w1299, length=w1291, index (col)=0 ("disabled index (col)")) -> (deleted portion=w1294:i8[], array with subset deleted=w1290:i8[][])  [unwired: 1 in]
                    n527 = for {
                      tunnel: w1294 -> [w1302] mode=indexing
                      tunnel: [w1301] -> w1293 mode=indexing
                      n528 = call-poly <vilib>:"Mean.vi"("X"=w1302) -> ("mean"=w1303:dbl)  [unwired: 1 out]
                      n529 = To Word Integer(number=w1303) -> (16bit integer=w1300:i16)
                      n530 = Subtract(x=w1302, y=w1300) -> (x-y=w1301:i16)
                    }
                    n531 = call-poly "TimeShiftDataPoly.vi"("output cluster"=w1298, "Array In"=w1293) -> ("Array Out"=w1297:i16[][])  [unwired: 2 in]
                    n532 = in-place {
                      in-place-border: w1297 -> [w1306]
                      n533 = in-place-dvr #7(w1295) -> (w1304:i16[][])  [unwired: 1 out]
                      n534 = Add(x=w1306, y=w1304) -> (x+y=w1305:i16[][])
                      n535 = in-place-dvr #7(w1305) -> (w1296:refnum<data-value>)  [unwired: 1 out]
                    }
                  }
                }
                n536 = local write "SF Index"(w1261) -> ()
                n537 = local read "stop out"() -> (w1262:bool)
                n538 = Or Array Elements(Boolean array=w1252) -> (logical OR=w1253:bool)
                n539 = in-place {
                  in-place-border: w1264 -> [w1274]
                  in-place-border: w1253 -> [w1273]
                  in-place-border: w1263 -> [w1272]
                  n540 = in-place-dvr #8(w1259) -> (w1268:i16[][])  [unwired: 1 out]
                  n541 = Bundle("gain"=w1272, w1273, w1268) -> (w1271:cluster{"gain":dbl, bool, i16[][]})  [unwired: 1 in]
                  n542 = Multiply(x=i16 0, y=w1268) -> (x*y=w1270:i16[][])
                  n543 = Enqueue Element(queue=w1274, element=w1271) -> ()  [unwired: 2 in, 3 out]
                  n544 = in-place-dvr #8(w1270) -> (w1251:refnum<data-value>)  [unwired: 1 out]
                }
                n545 = Tick Count (ms)() -> (millisecond timer value=w1257:u32)
                n546 = Subtract(x=w1257, y=w1258) -> (x-y=w1256:u32)
              }
              n547 = while {
                tunnel: w1231 -> [w1372]
                tunnel: w1228 -> [w1366]
                tunnel: [w1369] -> _
                tunnel: [w1371] -> w1232
                i -> [w1373]
                stop <- w1369 stop-if-true
                # "Slightly faster version to read data"
                # "Get and display data"
                n548 = Dequeue Element(queue=w1366, timeout in ms (-1)=5000) -> (queue out=w1371:refnum<queue>, element=w1368:cluster{"gain":dbl, bool, "wfm":i16[][]})  [unwired: 1 in, 2 out]
                n549 = Unbundle(w1368) -> ("gain"=w1363:dbl, w1364:bool, "wfm"=w1365:i16[][])
                n550 = case shown="True" w1364 {
                  tunnel: w1365 -> [w1374 w1376]
                  tunnel: [w1374 w1375] -> w1367
                  frame False {
                  }
                  frame True {
                    n551 = call "ReverseData.vi"("Array in"=w1376) -> ("Array out"=w1375:i16[][])
                  }
                }
                n552 = Increment(x=w1373) -> (x+1=w1362:i32)
                n553 = local write "Display index"(w1362) -> ()
                n554 = call "CurrentPlane.vi"("gain"=w1363, "bits A/D"=13, "Axis Vals"=w1372, "Frame"=w1362, "Data"=w1367) -> ("stop out"=w1369:bool)  [unwired: 5 in, 1 out]
                n555 = local write "stop out"(w1369) -> ()
              }
              n556 = Delete Data Value Reference(data value reference=w1220) -> ()  [unwired: 1 in, 2 out]
              n557 = Release Queue(queue=w1234, force destroy? (F)=w1233) -> ()  [unwired: 1 in, 3 out]
              n558 = Release Queue(queue=w1232, force destroy? (F)=w1233) -> ()  [unwired: 1 in, 3 out]
            }
            frame 6 {
              w1387 = 5
              # "Not fast enough for read"
              # "Read queue and send to files for chans 1,2"
              n559 = Reshape Array(w1382, w1387, w1387) -> (w1383:T12)
              n560 = Initialize Array(i16 0, w1392, w1378) -> (w1394:i16[][])
              n561 = Array Subset(array=w1383, length (col)=2 ("index")) -> (w1384:T12)  [unwired: 3 in]
              n562 = Obtain Queue(max queue size (-1, unlimited)=30, element data type=cluster{"gain":dbl, "wfm":i8[][], bool} {"gain"=0.0, "wfm"=[], TRUE}) -> (queue out=w1389:refnum<queue>)  [unwired: 3 in, 2 out]
              n563 = New Data Value Reference(data value=w1394) -> (data value reference=w1393:refnum<data-value>)  [unwired: 1 in, 1 out]
              n564 = Reshape Array(w1384, 10) -> (w1381:T13)
              n565 = Obtain Queue(max queue size (-1, unlimited)=3, element data type=cluster{"gain":dbl, bool, "wfm":i16[][]} {"gain"=0.0, TRUE, "wfm"=[]}) -> (queue out=w1395:refnum<queue>)  [unwired: 3 in, 2 out]
              n566 = Tick Count (ms)() -> (millisecond timer value=w1388:u32)
              n567 = while {
                tunnel: w1392 -> [w1453]
                tunnel: w1378 -> [w1452]
                tunnel: w1391 -> [w1449]
                tunnel: w1389 -> [w1448]
                shift-right: [w1444] -> _
                shift-left: w1388 -> [w1446]
                tunnel: [w1445] -> _
                tunnel: w1379 -> [w1443]
                i -> [w1450]
                stop <- w1451 stop-if-true
                # "Read files and queue it up."
                # "Read data"
                n568 = local write "Read Data index"(w1450) -> ()
                n569 = call "Rapid Read_2Ch.vi"("NI Card 3"=w1443, "Motion Board ID"=w1449, "rf points per line"=w1452, "lines per plane"=w1453, "queue out"=w1448) -> ("error out"=w1447:errorcluster)  [unwired: 7 in, 3 out]
                n570 = flat-sequence {
                  tunnel: w1447 -> [_]
                  tunnel: [w1454] -> w1444
                  frame #0 {
                    n571 = Tick Count (ms)() -> (millisecond timer value=w1454:u32)
                  }
                }
                n572 = local read "stop out"() -> (w1451:bool)
                n573 = Subtract(x=w1444, y=w1446) -> (x-y=w1445:u32)
              }
              n574 = while {
                tunnel: w1389 -> [w1407]
                tunnel: w1381 -> [w1415]
                tunnel: [w1411] -> w1399
                tunnel: w1393 -> [w1409]
                tunnel: w1395 -> [w1414]
                tunnel: [w1407] -> w1390
                tunnel: i16[] [1, 1, 1, 1, 2, 2, 2, 2, 2, 2] -> [w1406]
                tunnel: [w1405] -> w1377
                i -> [w1410]
                stop <- w1411 stop-if-true
                n575 = for {
                  tunnel: w1407 -> [w1433]
                  tunnel: w1415 -> [w1425] mode=indexing
                  tunnel: [w1430] -> w1413
                  tunnel: [w1429] -> w1412
                  tunnel: [w1428] -> w1408
                  tunnel: w1409 -> [w1427]
                  tunnel: w1406 -> [w1423] mode=indexing
                  n576 = Dequeue Element(queue=w1433, timeout in ms (-1)=10000) -> (element=w1432:cluster{"gain":dbl, "wfm":i8[][], bool})  [unwired: 1 in, 3 out]
                  n577 = Unbundle(w1432) -> ("gain"=w1429:dbl, "wfm"=w1424:i8[][], w1430:bool)
                  n578 = call-poly "TimeShiftDataPoly.vi"("output cluster"=w1425, "Array In"=w1424) -> ("Array Out"=w1426:i8[][])  [unwired: 1 in, 1 out]
                  n579 = in-place {
                    in-place-border: w1426 -> [w1435]
                    in-place-border: w1423 -> [w1436]
                    n580 = in-place-dvr #9(w1427) -> (w1437:i16[][])  [unwired: 1 out]
                    n581 = case shown="2" w1436 {
                      selector: w1436 -> [_ w1440]
                      tunnel: w1435 -> [w1439 w1442]
                      tunnel: [w1439 w1441] -> w1434
                      frame 0, Default {
                      }
                      frame 2 {
                        n582 = Multiply(x=w1440, y=w1442) -> (x*y=w1441:i16[][])
                      }
                    }
                    n583 = Add(x=w1434, y=w1437) -> (x+y=w1438:i16[][])
                    n584 = in-place-dvr #9(w1438) -> (w1428:refnum<data-value>)  [unwired: 1 out]
                  }
                }
                n585 = local write "SF Index"(w1410) -> ()
                n586 = local read "stop out"() -> (w1411:bool)
                n587 = in-place {
                  in-place-border: w1414 -> [w1422]
                  in-place-border: w1413 -> [w1421]
                  in-place-border: w1412 -> [w1420]
                  n588 = in-place-dvr #10(w1408) -> (w1416:i16[][])  [unwired: 1 out]
                  n589 = Bundle("gain"=w1420, w1421, w1416) -> (w1419:cluster{"gain":dbl, bool, i16[][]})  [unwired: 1 in]
                  n590 = Multiply(x=i16 0, y=w1416) -> (x*y=w1418:i16[][])
                  n591 = Enqueue Element(queue=w1422, element=w1419) -> ()  [unwired: 2 in, 3 out]
                  n592 = in-place-dvr #10(w1418) -> (w1405:refnum<data-value>)  [unwired: 1 out]
                }
              }
              n593 = while {
                tunnel: w1397 -> [w1466]
                tunnel: w1395 -> [w1460]
                tunnel: [w1463] -> _
                tunnel: [w1465] -> w1398
                i -> [w1467]
                stop <- w1463 stop-if-true
                # "Slightly faster version to read data"
                # "Get and display data"
                n594 = Dequeue Element(queue=w1460, timeout in ms (-1)=3000) -> (queue out=w1465:refnum<queue>, element=w1462:cluster{"gain":dbl, bool, "wfm":i16[][]})  [unwired: 1 in, 2 out]
                n595 = Unbundle(w1462) -> ("gain"=w1457:dbl, w1458:bool, "wfm"=w1459:i16[][])
                n596 = case shown="True" w1458 {
                  tunnel: w1459 -> [w1468 w1470]
                  tunnel: [w1468 w1469] -> w1461
                  frame False {
                  }
                  frame True {
                    n597 = call "ReverseData.vi"("Array in"=w1470) -> ("Array out"=w1469:i16[][])
                  }
                }
                n598 = Increment(x=w1467) -> (x+1=w1456:i32)
                n599 = local write "Display index"(w1456) -> ()
                n600 = call "CurrentPlane.vi"("gain"=w1457, "bits A/D"=13, "Axis Vals"=w1466, "Frame"=w1456, "Data"=w1461) -> ("stop out"=w1463:bool)  [unwired: 5 in, 1 out]
                n601 = local write "stop out"(w1463) -> ()
              }
              n602 = Release Queue(queue=w1398, force destroy? (F)=w1399) -> ()  [unwired: 1 in, 3 out]
              n603 = Delete Data Value Reference(data value reference=w1377) -> ()  [unwired: 1 in, 2 out]
              n604 = Release Queue(queue=w1390, force destroy? (F)=w1399) -> ()  [unwired: 1 in, 3 out]
            }
            frame 7 {
              # "Not fast enough for read"
              # "Read queue and send to files all 25"
              n605 = global read "MotionGlobals.vi" "rf points per line"() -> (w1482)
              n606 = Initialize Array(i16 0, w1477, w1482) -> (w1480:i16[][])
              n607 = Obtain Queue(max queue size (-1, unlimited)=75, element data type=cluster{"gain":dbl, "wfm":i8[][], bool} {"gain"=0.0, "wfm"=[], TRUE}) -> (queue out=w1474:refnum<queue>)  [unwired: 3 in, 2 out]
              n608 = New Data Value Reference(data value=w1480) -> (data value reference=w1479:refnum<data-value>)  [unwired: 1 in, 1 out]
              n609 = Tick Count (ms)() -> (millisecond timer value=w1473:u32)
              n610 = Obtain Queue(max queue size (-1, unlimited)=3, element data type=cluster{"gain":dbl, bool, "wfm":i16[][]} {"gain"=0.0, TRUE, "wfm"=[]}) -> (queue out=w1481:refnum<queue>)  [unwired: 3 in, 2 out]
              n611 = while {
                tunnel: w1477 -> [w1533]
                tunnel: w1490 -> [w1532]
                tunnel: w1471 -> [w1529]
                tunnel: w1476 -> [w1528]
                tunnel: w1474 -> [w1527]
                tunnel: [w1526] -> _
                shift-right: [w1523] -> _
                shift-left: w1473 -> [w1525]
                tunnel: [w1524] -> _
                i -> [w1530]
                stop <- w1531 stop-if-true
                # "Read files and queue it up."
                # "Read data"
                n612 = local write "Read Data index"(w1530) -> ()
                n613 = call "Rapid Read_5Ch.vi"("Dig Cards"=w1529, "Motion Board ID"=w1528, "rf points per line"=w1532, "lines per plane"=w1533, "queue out"=w1527) -> ("error out"=w1526:errorcluster)  [unwired: 7 in, 3 out]
                n614 = flat-sequence {
                  tunnel: w1526 -> [_]
                  tunnel: [w1534] -> w1523
                  frame #0 {
                    n615 = Tick Count (ms)() -> (millisecond timer value=w1534:u32)
                  }
                }
                n616 = local read "stop out"() -> (w1531:bool)
                n617 = Subtract(x=w1523, y=w1525) -> (x-y=w1524:u32)
              }
              n618 = while {
                tunnel: w1474 -> [w1494]
                tunnel: w1478 -> [w1502]
                tunnel: [w1498] -> w1486
                tunnel: w1479 -> [w1496]
                tunnel: w1481 -> [w1501]
                tunnel: [w1494] -> w1475
                tunnel: [w1493] -> w1472
                i -> [w1497]
                stop <- w1498 stop-if-true
                n619 = for {
                  tunnel: w1494 -> [w1519]
                  tunnel: w1502 -> [w1511] mode=indexing
                  tunnel: [w1516] -> w1500
                  tunnel: [w1515] -> w1499
                  tunnel: [w1514] -> w1495
                  tunnel: w1496 -> [w1513]
                  n620 = Dequeue Element(queue=w1519, timeout in ms (-1)=10000) -> (element=w1518:cluster{"gain":dbl, "wfm":i8[][], bool})  [unwired: 1 in, 3 out]
                  n621 = Unbundle(w1518) -> ("gain"=w1515:dbl, "wfm"=w1510:i8[][], w1516:bool)
                  n622 = call-poly "TimeShiftDataPoly.vi"("output cluster"=w1511, "Array In"=w1510) -> ("Array Out"=w1512:i8[][])  [unwired: 1 in, 1 out]
                  n623 = in-place {
                    in-place-border: w1512 -> [w1522]
                    n624 = in-place-dvr #11(w1513) -> (w1520:i16[][])  [unwired: 1 out]
                    n625 = Add(x=w1522, y=w1520) -> (x+y=w1521:i16[][])
                    n626 = in-place-dvr #11(w1521) -> (w1514:refnum<data-value>)  [unwired: 1 out]
                  }
                }
                n627 = local write "SF Index"(w1497) -> ()
                n628 = local read "stop out"() -> (w1498:bool)
                n629 = in-place {
                  in-place-border: w1501 -> [w1509]
                  in-place-border: w1500 -> [w1508]
                  in-place-border: w1499 -> [w1507]
                  n630 = in-place-dvr #12(w1495) -> (w1503:i16[][])  [unwired: 1 out]
                  n631 = Bundle("gain"=w1507, w1508, w1503) -> (w1506:cluster{"gain":dbl, bool, i16[][]})  [unwired: 1 in]
                  n632 = Multiply(x=i16 0, y=w1503) -> (x*y=w1505:i16[][])
                  n633 = Enqueue Element(queue=w1509, element=w1506) -> ()  [unwired: 2 in, 3 out]
                  n634 = in-place-dvr #12(w1505) -> (w1493:refnum<data-value>)  [unwired: 1 out]
                }
              }
              n635 = while {
                tunnel: w1484 -> [w1546]
                tunnel: w1481 -> [w1540]
                tunnel: [w1543] -> _
                tunnel: [w1545] -> w1485
                i -> [w1547]
                stop <- w1543 stop-if-true
                # "Slightly faster version to read data"
                # "Get and display data"
                n636 = Dequeue Element(queue=w1540, timeout in ms (-1)=3000) -> (queue out=w1545:refnum<queue>, element=w1542:cluster{"gain":dbl, bool, "wfm":i16[][]})  [unwired: 1 in, 2 out]
                n637 = Unbundle(w1542) -> ("gain"=w1537:dbl, w1538:bool, "wfm"=w1539:i16[][])
                n638 = case shown="True" w1538 {
                  tunnel: w1539 -> [w1548 w1550]
                  tunnel: [w1548 w1549] -> w1541
                  frame False {
                  }
                  frame True {
                    n639 = call "ReverseData.vi"("Array in"=w1550) -> ("Array out"=w1549:i16[][])
                  }
                }
                n640 = Increment(x=w1547) -> (x+1=w1536:i32)
                n641 = local write "Display index"(w1536) -> ()
                n642 = call "CurrentPlane.vi"("gain"=w1537, "bits A/D"=13, "Axis Vals"=w1546, "Frame"=w1536, "Data"=w1541) -> ("stop out"=w1543:bool)  [unwired: 5 in, 1 out]
                n643 = local write "stop out"(w1543) -> ()
              }
              n644 = Release Queue(queue=w1475, force destroy? (F)=w1486) -> ()  [unwired: 1 in, 3 out]
              n645 = Release Queue(queue=w1485, force destroy? (F)=w1486) -> ()  [unwired: 1 in, 3 out]
              n646 = Delete Data Value Reference(data value reference=w1472) -> ()  [unwired: 1 in, 2 out]
            }
            frame 8 {
              w1572 = 5
              # "Just Ch 1,2. Also cam suffer memory overflow if Byte depth too small"
              # "Arm digitizer"
              n647 = Reshape Array(w1567, w1572, w1572) -> (w1568:T12)
              n648 = call <instrlib>:"niScope Initiate Acquisition.vi"("instrument handle"=w1582) -> ("error out"=w1554:errorcluster)  [unwired: 2 in, 12 out]
              n649 = expression code="x*5"(w1558) -> (w1573:dbl)
              n650 = Initialize Array(i16 0, w1558, w1561) -> (w1580:i16[][])
              n651 = Array Subset(array=w1568, length (col)=2 ("index")) -> (w1569:T12)  [unwired: 3 in]
              n652 = Tick Count (ms)() -> (millisecond timer value=w1551:u32)
              n653 = Obtain Queue(max queue size (-1, unlimited)=5, element data type=cluster{"Fetch:Records Done":i32, bool} {"Fetch:Records Done"=0, TRUE}) -> (queue out=w1552:refnum<queue>)  [unwired: 2 in, 3 out]
              n654 = node-c288(i64 50 ("Period")) -> (w1584:T6)
              n655 = Obtain Queue(max queue size (-1, unlimited)=5, element data type=i8[][] [] ("Array")) -> (queue out=w1566:refnum<queue>)  [unwired: 2 in, 3 out]
              n656 = New Data Value Reference(data value=w1580) -> (data value reference=w1564:refnum<data-value>)  [unwired: 1 in, 1 out]
              n657 = Tick Count (ms)() -> (millisecond timer value=w1560:u32)
              n658 = Obtain Queue(max queue size (-1, unlimited)=5, element data type=i16[][] [] ("wfm")) -> (queue out=w1565:refnum<queue>)  [unwired: 3 in, 2 out]
              n659 = Reshape Array(w1569, 10) -> (w1563:T13)
              n660 = while {
                tunnel: w1552 -> [w1713]
                tunnel: [w1722] -> w1590
                tunnel: w1582 -> [w1723]
                tunnel: w1566 -> [w1725]
                tunnel: w1561 -> [w1714]
                tunnel: [w1709] -> w1588
                tunnel: w1554 -> [w1721]
                tunnel: w1573 -> [w1710]
                tunnel: [w1707] -> w1555
                shift-right: [w1706] -> _
                shift-left: w1551 -> [w1705]
                tunnel: [w1703] -> _
                i -> [w1716]
                stop <- w1722 stop-if-true
                # "This loop reads the data once it is in the queue"
                # "Get and display data"
                n661 = Dequeue Element(queue=w1713, timeout in ms (-1)=1000, error in (no error)=w1721) -> (queue out=w1712:refnum<queue>, element=w1726:cluster{"Fetch:Records Done":i32, bool}, error out=w1717:errorcluster)  [unwired: 1 out]
                n662 = Unbundle(w1726) -> ("Fetch:Records Done"=w1719:i32)  [unwired: 1 out]
                n663 = local write "Read Data index"(w1716) -> ()
                n664 = property class="niScope"(reference=w1723, error in=w1717, "Fetch Record Number"=w1719, "Fetch Number of Records"=w1710) -> (reference out=w1715:refnum<k15>, error out=w1718:errorcluster)
                n665 = call-poly <instrlib>:"niScope Fetch (poly).vi"("timeout"=3.0, "error in"=w1718, "numSamples"=w1714, "channels"="0,1", "instrument handle"=w1715) -> ("error out"=w1704:errorcluster, "wfm"=w1720:i8[][], "instrument handle out"=w1707:refnum<k15>)  [unwired: 4 out]
                n666 = case shown="No Error" w1704 {
                  tunnel: w1725 -> [w1733 w1734]
                  tunnel: w1720 -> [w1732 _]
                  tunnel: w1712 -> [w1731 _]
                  tunnel: [w1730 w1734] -> w1709
                  frame No Error {
                    n667 = Lossy Enqueue Element(queue=w1733, element=w1732) -> (queue out=w1730:refnum<queue>, error out=w1729:errorcluster)  [unwired: 1 in, 2 out]
                    n668 = Get Queue Status(queue=w1731, error in (no error)=w1729) -> (# elements in queue=w1728:i32)  [unwired: 1 in, 7 out]
                    n669 = local write "SF queue"(w1728) -> ()
                  }
                  frame Error {
                  }
                }
                n670 = stacked-sequence {
                  tunnel: [w1727] -> w1706
                  tunnel: w1704 -> [_]
                  frame #0 {
                    n671 = Tick Count (ms)() -> (millisecond timer value=w1727:u32)
                  }
                }
                n672 = Subtract(x=w1706, y=w1705) -> (x-y=w1703:u32)
                n673 = local read "stop out"() -> (w1722:bool)
              }
              n674 = timed-loop {
                shift-right: [w1671] -> _
                shift-left: 0 -> [w1678]
                shift-right: [w1684] -> _
                shift-left: TRUE -> [w1679]
                tunnel: w1593 -> [w1682]
                tunnel: [w1677] -> w1585
                tunnel: [w1667] -> w1589
                tunnel: w1582 -> [w1676]
                tunnel: w1586 -> [w1672]
                tunnel: w1554 -> [w1681]
                timing: w1584 -> [_]
                timing-out: [_] -> w1583
                tunnel: w1552 -> [w1664]
                i -> [w1666]
                stop <- w1677 stop-if-true
                # "This loop performs back and forth scan and records record # at end of run"
                n675 = Bundle(w1678, w1679) -> (w1675:cluster{i32, bool})  [unwired: 1 in]
                n676 = Select(t=T5 6 ("Program (1)"), s=w1679, f=T5 7 ("Program (1)")) -> (s? t:f=w1665:T5)
                n677 = call <vilib>:"Run Program.flx"("error in (no error)"=w1681, "Program (1)"=w1665, "Board ID"=w1682) -> ("error out"=w1674:errorcluster, "Bd ID Out"=w1669:T2)  [unwired: 4 out]
                n678 = stacked-sequence {
                  tunnel: w1674 -> [w1696]
                  tunnel: [w1696] -> w1673
                  tunnel: [w1694] -> w1670
                  tunnel: w1669 -> [w1694]
                  frame #0 {
                    n679 = Wait (ms)(milliseconds to wait=20) -> ()  [unwired: 1 out]
                  }
                }
                n680 = call-poly <vilib>:"Wait for Move Complete.flx"("Poll Interval (20 ms)"=5, "error in (no error)"=w1673, "Axis or Vector Space"=w1672, "Board ID"=w1670) -> ("error out"=w1680:errorcluster)  [unwired: 4 in, 3 out]
                n681 = property class="niScope"(reference=w1676, error in=w1680) -> (error out=w1663:errorcluster, "Records Done"=w1671:i32)  [unwired: 1 out]
                n682 = local write "Read Loop"(w1666) -> ()
                n683 = local read "stop out"() -> (w1677:bool)
                n684 = case shown="No Error" w1663 {
                  selector: w1663 -> [w1686 _]
                  tunnel: w1675 -> [w1692 _]
                  tunnel: [w1690 w1693] -> w1667
                  tunnel: w1664 -> [w1687 w1693]
                  frame No Error {
                    n685 = Lossy Enqueue Element(queue=w1687, element=w1692, error in (no error)=w1686) -> (queue out=w1691:refnum<queue>, error out=w1689:errorcluster)  [unwired: 2 out]
                    n686 = Get Queue Status(queue=w1691, error in (no error)=w1689) -> (queue out=w1690:refnum<queue>, # elements in queue=w1688:i32)  [unwired: 1 in, 6 out]
                    n687 = local write "Record queue"(w1688) -> ()
                  }
                  frame Error {
                  }
                }
                n688 = Not(x=w1679) -> (.not. x?=w1684:bool)
              }
              n689 = while {
                tunnel: w1566 -> [w1617]
                tunnel: w1558 -> [w1616]
                tunnel: w1564 -> [w1612]
                tunnel: w1565 -> [w1615]
                shift-right: [w1610] -> _
                shift-left: w1560 -> [w1611]
                tunnel: [w1609] -> _
                tunnel: w1563 -> [w1604]
                tunnel: i16[] [1, 1, 1, 1, 2, 2, 2, 2, 2, 2] -> [w1603]
                tunnel: 10 -> [w1602]
                tunnel: w1561 -> [w1601]
                tunnel: [w1599] -> w1557
                tunnel: w1554 -> [_]
                tunnel: [w1598] -> w1553
                i -> [w1613]
                stop <- w1614 stop-if-true
                n690 = local write "SF Index"(w1613) -> ()
                n691 = Dequeue Element(queue=w1617, timeout in ms (-1)=1000) -> (element=w1605:i8[][])  [unwired: 1 in, 3 out]
                n692 = Multiply(x=w1601, y=w1602) -> (x*y=w1606:i32)
                n693 = Reshape Array(w1605, w1616, w1606) -> (w1607:i8[][])
                n694 = for {
                  N: w1602 -> [_]
                  tunnel: w1604 -> [w1625]
                  tunnel: [w1628] -> w1608
                  tunnel: w1612 -> [w1627]
                  shift-right: [w1620] -> _
                  shift-left: w1607 -> [w1630]
                  tunnel: w1601 -> [w1619]
                  tunnel: w1603 -> [w1618] mode=indexing
                  i -> [w1626]
                  n695 = Index Array(array=w1625, index=w1626) -> (element=w1624:T11)
                  n696 = Delete From Array(array=w1630, length=w1619, index (col)=0 ("disabled index (col)")) -> (deleted portion=w1623:i8[], array with subset deleted=w1620:i8[][])  [unwired: 1 in]
                  n697 = for {
                    tunnel: w1623 -> [w1633] mode=indexing
                    tunnel: [w1632] -> w1622 mode=indexing
                    n698 = call-poly <vilib>:"Mean.vi"("X"=w1633) -> ("mean"=w1634:dbl)  [unwired: 1 out]
                    n699 = To Word Integer(number=w1634) -> (16bit integer=w1631:i16)
                    n700 = Subtract(x=w1633, y=w1631) -> (x-y=w1632:i16)
                  }
                  n701 = call-poly "TimeShiftDataPoly.vi"("output cluster"=w1624, "Array In"=w1622) -> ("Array Out"=w1629:i16[][])  [unwired: 2 in]
                  n702 = in-place {
                    in-place-border: w1629 -> [w1636]
                    in-place-border: w1618 -> [w1637]
                    n703 = in-place-dvr #13(w1627) -> (w1638:i16[][])  [unwired: 1 out]
                    n704 = case shown="2" w1637 {
                      selector: w1637 -> [_ w1641]
                      tunnel: w1636 -> [w1640 w1643]
                      tunnel: [w1640 w1642] -> w1635
                      frame 0, Default {
                      }
                      frame 2 {
                        n705 = Multiply(x=w1641, y=w1643) -> (x*y=w1642:i16[][])
                      }
                    }
                    n706 = Add(x=w1635, y=w1638) -> (x+y=w1639:i16[][])
                    n707 = in-place-dvr #13(w1639) -> (w1628:refnum<data-value>)  [unwired: 1 out]
                  }
                }
                n708 = local read "stop out"() -> (w1614:bool)
                n709 = in-place {
                  in-place-border: w1615 -> [w1648]
                  in-place-border: [w1644] -> w1599
                  n710 = in-place-dvr #14(w1608) -> (w1645:i16[][])  [unwired: 1 out]
                  n711 = Multiply(x=i16 0, y=w1645) -> (x*y=w1647:i16[][])
                  n712 = Enqueue Element(queue=w1648, element=w1645) -> (queue out=w1644:refnum<queue>)  [unwired: 2 in, 2 out]
                  n713 = in-place-dvr #14(w1647) -> (w1598:refnum<data-value>)  [unwired: 1 out]
                }
                n714 = Tick Count (ms)() -> (millisecond timer value=w1610:u32)
                n715 = Subtract(x=w1610, y=w1611) -> (x-y=w1609:u32)
              }
              n716 = while {
                tunnel: w1578 -> [w1658]
                tunnel: w1565 -> [w1654]
                tunnel: [w1656] -> w1577
                shift-right: [w1649] -> _
                shift-left: TRUE -> [w1650]
                tunnel: w1554 -> [_]
                i -> [w1659]
                stop <- w1656 stop-if-true
                # "Slightly faster version to read data"
                # "Get and display data"
                n717 = Dequeue Element(queue=w1654, timeout in ms (-1)=1000) -> (element=w1651:i16[][])  [unwired: 1 in, 3 out]
                n718 = case shown="True" w1650 {
                  tunnel: w1651 -> [w1660 w1662]
                  tunnel: [w1660 w1661] -> w1655
                  frame False {
                  }
                  frame True {
                    n719 = call "ReverseData.vi"("Array in"=w1662) -> ("Array out"=w1661:i16[][])
                  }
                }
                n720 = Not(x=w1650) -> (.not. x?=w1649:bool)
                n721 = Increment(x=w1659) -> (x+1=w1653:i32)
                n722 = local write "Display index"(w1653) -> ()
                n723 = call "CurrentPlane.vi"("bits A/D"=13, "Axis Vals"=w1658, "Frame"=w1653, "Data"=w1655) -> ("stop out"=w1656:bool)  [unwired: 6 in, 1 out]
                n724 = local write "stop out"(w1656) -> ()
              }
              n725 = node-c288(w1583) -> ()
              n726 = Compound Arithmetic op=AND(w1585, w1590, w1577) -> (w1574:bool)
              n727 = Release Queue(queue=w1589, force destroy? (F)=w1574) -> ()  [unwired: 1 in, 3 out]
              n728 = call <instrlib>:"niScope Abort.vi"("instrument handle"=w1555) -> ()  [unwired: 13 in, 2 out]
              n729 = Delete Data Value Reference(data value reference=w1553) -> ()  [unwired: 1 in, 2 out]
              n730 = Release Queue(queue=w1588, force destroy? (F)=w1574) -> ()  [unwired: 1 in, 3 out]
              n731 = Release Queue(queue=w1557, force destroy? (F)=w1574) -> ()  [unwired: 1 in, 3 out]
            }
            frame 9 {
              w1772 = 5
              # "Reduced data case that drop ring 4,5 receive"
              # "Restructure file names"
              # "Read queue and send to files. About same as reading channel by channel"
              n732 = Reshape Array(w1773, w1772, w1772) -> (w1745:T12)
              n733 = Initialize Array(i16 0, w1742, w1744) -> (w1762:i16[][])
              n734 = Array Subset(array=w1745, index (col)=2 ("index"), length (col)=1 ("index")) -> (w1746:T12)  [unwired: 2 in]
              n735 = Array Subset(array=w1745, length (col)=2 ("index")) -> (w1749:T12)  [unwired: 3 in]
              n736 = Obtain Queue(max queue size (-1, unlimited)=6, element data type=T9 {"gain"=0.0, "wfm"=[], TRUE, "max queue size (-1, unlimited)"=15}) -> (queue out=w1775:refnum<queue>)  [unwired: 3 in, 2 out]
              n737 = Build Array(w1741, w1739) -> (w1740:void[])
              n738 = New Data Value Reference(data value=w1762) -> (data value reference=w1761:refnum<data-value>)  [unwired: 1 in, 1 out]
              n739 = Reshape Array(w1749, 10) -> (w1748:T13)
              n740 = Reshape Array(w1746, 5) -> (w1759:T13)
              n741 = Obtain Queue(max queue size (-1, unlimited)=3, element data type=cluster{"gain":dbl, bool, "wfm":i16[][]} {"gain"=0.0, TRUE, "wfm"=[]}) -> (queue out=w1763:refnum<queue>)  [unwired: 3 in, 2 out]
              n742 = expression code="x*5"(w1742) -> (w1738:dbl)
              n743 = Tick Count (ms)() -> (millisecond timer value=w1756:u32)
              n744 = Build Array(w1748, w1759) -> (w1758:T12)
              n745 = while {
                tunnel: w1775 -> [w1796]
                tunnel: w1744 -> [w1795]
                tunnel: [w1791] -> w1767
                tunnel: w1742 -> [w1794]
                tunnel: w1761 -> [w1789]
                tunnel: w1763 -> [w1793]
                tunnel: w1758 -> [w1784]
                tunnel: i32[] [10, 5] -> [w1788]
                shift-right: [w1786] -> _
                shift-left: w1756 -> [w1787]
                tunnel: [w1785] -> _
                tunnel: 10000 -> [w1780]
                tunnel: i16[] [1, 1, 1, 1, 1, 1, 2, 2, 2, 2] -> [w1779]
                tunnel: [w1778] -> w1743
                tunnel: i16[] [1, 1, 1, 2, 2] -> [w1777]
                i -> [w1790]
                stop <- w1791 stop-if-true
                n746 = for {
                  tunnel: w1795 -> [w1810]
                  tunnel: w1794 -> [w1820]
                  tunnel: w1796 -> [w1823]
                  tunnel: [w1819] -> w1783 mode=indexing
                  tunnel: [w1818] -> w1792
                  tunnel: [w1817] -> w1781
                  tunnel: w1789 -> [w1816]
                  tunnel: w1784 -> [_] mode=indexing
                  tunnel: w1788 -> [w1813]
                  tunnel: w1784 -> [w1815]
                  tunnel: w1780 -> [w1812]
                  tunnel: w1779 -> [w1805]
                  tunnel: w1777 -> [w1804]
                  n747 = Dequeue Element(queue=w1823, timeout in ms (-1)=w1812) -> (element=w1822:T9)  [unwired: 1 in, 3 out]
                  n748 = Unbundle(w1822) -> ("gain"=w1818:dbl, "wfm"=w1821:i8[][], w1819:bool, "max queue size (-1, unlimited)"=w1807:i32)
                  n749 = Index Array(array=w1813, index=w1807) -> (element=w1811:i32)
                  n750 = Index Array(array=w1815, index (row)=w1807) -> (element=w1814:T13)  [unwired: 1 in]
                  n751 = case shown="1" w1807 {
                    tunnel: [w1824 w1825] -> w1806
                    tunnel: w1805 -> [w1824 _]
                    tunnel: w1804 -> [_ w1825]
                    frame 0, Default {
                    }
                    frame 1 {
                    }
                  }
                  n752 = Multiply(x=w1810, y=w1811) -> (x*y=w1809:i32)
                  n753 = Reshape Array(w1821, w1820, w1809) -> (w1808:i8[][])
                  n754 = for {
                    N: w1811 -> [_]
                    tunnel: w1814 -> [w1833]
                    tunnel: [w1836] -> w1817
                    tunnel: w1816 -> [w1835]
                    shift-right: [w1826] -> _
                    shift-left: w1808 -> [w1838]
                    tunnel: w1806 -> [w1828] mode=indexing
                    tunnel: w1810 -> [w1827]
                    i -> [w1834]
                    n755 = Index Array(array=w1833, index=w1834) -> (element=w1832:T11)
                    n756 = Delete From Array(array=w1838, length=w1827, index (col)=0 ("disabled index (col)")) -> (deleted portion=w1831:i8[], array with subset deleted=w1826:i8[][])  [unwired: 1 in]
                    n757 = for {
                      tunnel: w1831 -> [w1841] mode=indexing
                      tunnel: [w1840] -> w1830 mode=indexing
                      n758 = call-poly <vilib>:"Mean.vi"("X"=w1841) -> ("mean"=w1842:dbl)  [unwired: 1 out]
                      n759 = To Word Integer(number=w1842) -> (16bit integer=w1839:i16)
                      n760 = Subtract(x=w1841, y=w1839) -> (x-y=w1840:i16)
                    }
                    n761 = call-poly "TimeShiftDataPoly.vi"("output cluster"=w1832, "Array In"=w1830) -> ("Array Out"=w1837:i16[][])  [unwired: 2 in]
                    n762 = in-place {
                      in-place-border: w1837 -> [w1844]
                      in-place-border: w1828 -> [w1845]
                      n763 = in-place-dvr #15(w1835) -> (w1846:i16[][])  [unwired: 1 out]
                      n764 = case shown="2" w1845 {
                        selector: w1845 -> [_ w1849]
                        tunnel: w1844 -> [w1848 w1851]
                        tunnel: [w1848 w1850] -> w1843
                        frame 0, Default {
                        }
                        frame 2 {
                          n765 = Multiply(x=w1849, y=w1851) -> (x*y=w1850:i16[][])
                        }
                      }
                      n766 = Add(x=w1843, y=w1846) -> (x+y=w1847:i16[][])
                      n767 = in-place-dvr #15(w1847) -> (w1836:refnum<data-value>)  [unwired: 1 out]
                    }
                  }
                }
                n768 = local write "SF Index"(w1790) -> ()
                n769 = local read "stop out"() -> (w1791:bool)
                n770 = Or Array Elements(Boolean array=w1783) -> (logical OR=w1782:bool)
                n771 = in-place {
                  in-place-border: w1793 -> [w1803]
                  in-place-border: w1782 -> [w1802]
                  in-place-border: w1792 -> [w1801]
                  n772 = in-place-dvr #16(w1781) -> (w1797:i16[][])  [unwired: 1 out]
                  n773 = Bundle("gain"=w1801, w1802, w1797) -> (w1800:cluster{"gain":dbl, bool, i16[][]})  [unwired: 1 in]
                  n774 = Multiply(x=i16 0, y=w1797) -> (x*y=w1799:i16[][])
                  n775 = Enqueue Element(queue=w1803, element=w1800) -> ()  [unwired: 2 in, 3 out]
                  n776 = in-place-dvr #16(w1799) -> (w1778:refnum<data-value>)  [unwired: 1 out]
                }
                n777 = Tick Count (ms)() -> (millisecond timer value=w1786:u32)
                n778 = Subtract(x=w1786, y=w1787) -> (x-y=w1785:u32)
              }
              n779 = while {
                tunnel: w1765 -> [w1915]
                tunnel: w1763 -> [w1909]
                tunnel: [w1912] -> _
                tunnel: [w1914] -> w1766
                i -> [w1916]
                stop <- w1912 stop-if-true
                # "Slightly faster version to read data"
                # "Get and display data"
                n780 = Dequeue Element(queue=w1909, timeout in ms (-1)=5000) -> (queue out=w1914:refnum<queue>, element=w1911:cluster{"gain":dbl, bool, "wfm":i16[][]})  [unwired: 1 in, 2 out]
                n781 = Unbundle(w1911) -> ("gain"=w1906:dbl, w1907:bool, "wfm"=w1908:i16[][])
                n782 = case shown="False" w1907 {
                  tunnel: w1908 -> [w1917 w1919]
                  tunnel: [w1917 w1918] -> w1910
                  frame False {
                  }
                  frame True {
                    n783 = call "ReverseData.vi"("Array in"=w1919) -> ("Array out"=w1918:i16[][])
                  }
                }
                n784 = Increment(x=w1916) -> (x+1=w1905:i32)
                n785 = local write "Display index"(w1905) -> ()
                n786 = call "CurrentPlane.vi"("gain"=w1906, "bits A/D"=13, "Axis Vals"=w1915, "Frame"=w1905, "Data"=w1910) -> ("stop out"=w1912:bool)  [unwired: 5 in, 1 out]
                n787 = local write "stop out"(w1912) -> ()
              }
              n788 = global read "MotionGlobals.vi" "DigTimeOut"() -> (w1755)
              n789 = while {
                tunnel: w1740 -> [w1864]
                tunnel: w1775 -> [w1863]
                tunnel: w1739 -> [w1862]
                tunnel: w1744 -> [w1861]
                tunnel: [w1860] -> w1768
                tunnel: w1760 -> [w1858]
                shift-right: [w1856] -> _
                shift-left: w1756 -> [w1857]
                tunnel: [w1855] -> _
                tunnel: w1755 -> [w1854]
                tunnel: "0,1" -> [w1853]
                tunnel: w1738 -> [w1852]
                stop <- w1859 stop-if-true
                n790 = for {
                  tunnel: w1861 -> [w1877]
                  tunnel: w1864 -> [w1879] mode=indexing
                  tunnel: w1853 -> [w1878]
                  tunnel: w1863 -> [w1876]
                  tunnel: [w1872] -> _
                  tunnel: w1862 -> [w1871]
                  tunnel: [w1869] -> w1860
                  tunnel: w1858 -> [w1868]
                  tunnel: w1854 -> [w1867]
                  tunnel: w1852 -> [w1865]
                  i -> [w1866]
                  # "Read data"
                  n791 = case shown="1, Default" w1866 {
                    tunnel: w1879 -> [w1886 w1895]
                    tunnel: w1878 -> [w1884 _]
                    tunnel: w1877 -> [w1887 w1900]
                    tunnel: [w1888 w1899] -> w1875
                    tunnel: [w1881 w1894] -> w1874
                    tunnel: [w1889 w1898] -> w1872
                    tunnel: w1871 -> [w1890 _]
                    tunnel: [w1885 _] -> w1870
                    tunnel: w1868 -> [w1883 _]
                    tunnel: w1867 -> [_ w1896]
                    tunnel: w1865 -> [w1880 w1892]
                    frame 0 {
                      # "Read files and queue it up."
                      n792 = call <instrlib>:"niScope Initiate Acquisition.vi"("instrument handle"=w1890) -> ("error out"=w1882:errorcluster)  [unwired: 2 in, 12 out]
                      n793 = call "Rapid Read_NI.vi"("Channel"=w1884, "lines per plane"=w1880, "error in"=w1882, "rf points per line"=w1887, "Motion Board ID"=w1883, "NI Card"=w1886) -> ("error out"=w1889:errorcluster, "Reverse?"=w1885:bool, "Array"=w1881:i8[][], "dig gain"=w1888:dbl)  [unwired: 2 in]
                    }
                    frame 1, Default {
                      n794 = property class="niScope"(reference=w1895, "Fetch Record Number"=0, "Fetch Number of Records"=w1892) -> (reference out=w1901:refnum<k15>, error out=w1897:errorcluster)  [unwired: 1 in]
                      n795 = call-poly <instrlib>:"niScope Fetch (poly).vi"("timeout"=w1896, "error in"=w1897, "numSamples"=w1900, "channels"="0", "instrument handle"=w1901) -> ("error out"=w1898:errorcluster, "wfm"=w1894:i8[][], "wfm info"=w1903:T14)  [unwired: 4 out]
                      n796 = Index Array(array=w1903) -> (element=w1902:T15)  [unwired: 1 in]
                      n797 = Unbundle By Name(w1902) -> ("gain"=w1899:dbl)
                    }
                  }
                  n798 = local write "Read Data index"(w1866) -> ()
                  n799 = Bundle("gain"=w1875, "wfm"=w1874, "Reverse?"=w1870, w1866) -> (w1873:T16)  [unwired: 1 in]
                  n800 = Enqueue Element(queue=w1876, element=w1873) -> (queue out=w1869:refnum<queue>)  [unwired: 2 in, 2 out]
                }
                n801 = local read "stop out"() -> (w1859:bool)
                n802 = Tick Count (ms)() -> (millisecond timer value=w1856:u32)
                n803 = Subtract(x=w1856, y=w1857) -> (x-y=w1855:u32)
              }
              n804 = Release Queue(queue=w1768, force destroy? (F)=w1767) -> ()  [unwired: 1 in, 3 out]
              n805 = Release Queue(queue=w1766, force destroy? (F)=w1767) -> ()  [unwired: 1 in, 3 out]
              n806 = Delete Data Value Reference(data value reference=w1743) -> ()  [unwired: 1 in, 2 out]
            }
            frame 10 {
              w1932 = 2 ("index")
              w1957 = 5
              # "Reduced data case that drop ring 5 receive using rcv on 3,4,5"
              # "Restructure file names"
              # "Read queue and send to files. About same as reading channel by channel"
              n807 = Reshape Array(w1958, w1957, w1957) -> (w1930:T12)
              n808 = Initialize Array(i16 0, w1921, w1929) -> (w1947:i16[][])
              n809 = Array Subset(array=w1930, index (row)=2 ("index"), index (col)=w1932, length (col)=w1932) -> (w1931:T12)  [unwired: 1 in]
              n810 = Array Subset(array=w1930, length (col)=2 ("index")) -> (w1934:T12)  [unwired: 3 in]
              n811 = Obtain Queue(max queue size (-1, unlimited)=6, element data type=T9 {"gain"=0.0, "wfm"=[], TRUE, "max queue size (-1, unlimited)"=15}) -> (queue out=w1960:refnum<queue>)  [unwired: 3 in, 2 out]
              n812 = Build Array(w1927, w1925) -> (w1926:void[])
              n813 = New Data Value Reference(data value=w1947) -> (data value reference=w1946:refnum<data-value>)  [unwired: 1 in, 1 out]
              n814 = Reshape Array(w1934, 10) -> (w1933:T13)
              n815 = Reshape Array(w1931, 6) -> (w1944:T13)
              n816 = Obtain Queue(max queue size (-1, unlimited)=3, element data type=cluster{"gain":dbl, bool, "wfm":i16[][]} {"gain"=0.0, TRUE, "wfm"=[]}) -> (queue out=w1948:refnum<queue>)  [unwired: 3 in, 2 out]
              n817 = expression code="x*5"(w1921) -> (w1924:dbl)
              n818 = expression code="x*3"(w1921) -> (w1920:dbl)
              n819 = Tick Count (ms)() -> (millisecond timer value=w1941:u32)
              n820 = Build Array(w1933, w1944) -> (w1943:T12)
              n821 = while {
                tunnel: w1960 -> [w1980]
                tunnel: w1929 -> [w1979]
                tunnel: [w1975] -> w1952
                tunnel: w1921 -> [w1978]
                tunnel: w1946 -> [w1973]
                tunnel: w1948 -> [w1977]
                tunnel: w1943 -> [w1968]
                tunnel: i32[] [10, 6] -> [w1972]
                shift-right: [w1970] -> _
                shift-left: w1941 -> [w1971]
                tunnel: [w1969] -> _
                tunnel: 10000 -> [w1964]
                tunnel: i16[] [1, 1, 1, 1, 2, 2, 2, 2, 2, 2] -> [w1963]
                tunnel: [w1962] -> w1928
                i -> [w1974]
                stop <- w1975 stop-if-true
                n822 = for {
                  tunnel: w1979 -> [w1991]
                  tunnel: w1978 -> [w2002]
                  tunnel: w1980 -> [w2005]
                  tunnel: [w2001] -> w1967 mode=indexing
                  tunnel: [w2000] -> w1976
                  tunnel: [w1999] -> w1965
                  tunnel: w1973 -> [w1998]
                  tunnel: w1968 -> [_] mode=indexing
                  tunnel: w1972 -> [w1995]
                  tunnel: w1968 -> [w1997]
                  tunnel: w1964 -> [w1994]
                  tunnel: w1963 -> [w1990]
                  n823 = Dequeue Element(queue=w2005, timeout in ms (-1)=w1994) -> (element=w2004:T9)  [unwired: 1 in, 3 out]
                  n824 = Unbundle(w2004) -> ("gain"=w2000:dbl, "wfm"=w2003:i8[][], w2001:bool, "max queue size (-1, unlimited)"=w1992:i32)
                  n825 = Index Array(array=w1995, index=w1992) -> (element=w1993:i32)
                  n826 = Index Array(array=w1997, index (row)=w1992) -> (element=w1996:T13)  [unwired: 1 in]
                  n827 = Multiply(x=w1991, y=w1993) -> (x*y=w1989:i32)
                  n828 = Reshape Array(w2003, w2002, w1989) -> (w1988:i8[][])
                  n829 = for {
                    N: w1993 -> [_]
                    tunnel: w1996 -> [w2013]
                    tunnel: [w2016] -> w1999
                    tunnel: w1998 -> [w2015]
                    shift-right: [w2006] -> _
                    shift-left: w1988 -> [w2018]
                    tunnel: w1990 -> [w2008] mode=indexing
                    tunnel: w1991 -> [w2007]
                    i -> [w2014]
                    n830 = Index Array(array=w2013, index=w2014) -> (element=w2012:T11)
                    n831 = Delete From Array(array=w2018, length=w2007, index (col)=0 ("disabled index (col)")) -> (deleted portion=w2011:i8[], array with subset deleted=w2006:i8[][])  [unwired: 1 in]
                    n832 = for {
                      tunnel: w2011 -> [w2021] mode=indexing
                      tunnel: [w2020] -> w2010 mode=indexing
                      n833 = call-poly <vilib>:"Mean.vi"("X"=w2021) -> ("mean"=w2022:dbl)  [unwired: 1 out]
                      n834 = To Word Integer(number=w2022) -> (16bit integer=w2019:i16)
                      n835 = Subtract(x=w2021, y=w2019) -> (x-y=w2020:i16)
                    }
                    n836 = call-poly "TimeShiftDataPoly.vi"("output cluster"=w2012, "Array In"=w2010) -> ("Array Out"=w2017:i16[][])  [unwired: 2 in]
                    n837 = in-place {
                      in-place-border: w2017 -> [w2024]
                      in-place-border: w2008 -> [w2025]
                      n838 = in-place-dvr #17(w2015) -> (w2026:i16[][])  [unwired: 1 out]
                      n839 = case shown="2" w2025 {
                        selector: w2025 -> [_ w2029]
                        tunnel: w2024 -> [w2028 w2031]
                        tunnel: [w2028 w2030] -> w2023
                        frame 0, Default {
                        }
                        frame 2 {
                          n840 = Multiply(x=w2029, y=w2031) -> (x*y=w2030:i16[][])
                        }
                      }
                      n841 = Add(x=w2023, y=w2026) -> (x+y=w2027:i16[][])
                      n842 = in-place-dvr #17(w2027) -> (w2016:refnum<data-value>)  [unwired: 1 out]
                    }
                  }
                }
                n843 = local write "SF Index"(w1974) -> ()
                n844 = local read "stop out"() -> (w1975:bool)
                n845 = Or Array Elements(Boolean array=w1967) -> (logical OR=w1966:bool)
                n846 = in-place {
                  in-place-border: w1977 -> [w1987]
                  in-place-border: w1966 -> [w1986]
                  in-place-border: w1976 -> [w1985]
                  n847 = in-place-dvr #18(w1965) -> (w1981:i16[][])  [unwired: 1 out]
                  n848 = Bundle("gain"=w1985, w1986, w1981) -> (w1984:cluster{"gain":dbl, bool, i16[][]})  [unwired: 1 in]
                  n849 = Multiply(x=i16 0, y=w1981) -> (x*y=w1983:i16[][])
                  n850 = Enqueue Element(queue=w1987, element=w1984) -> ()  [unwired: 2 in, 3 out]
                  n851 = in-place-dvr #18(w1983) -> (w1962:refnum<data-value>)  [unwired: 1 out]
                }
                n852 = Tick Count (ms)() -> (millisecond timer value=w1970:u32)
                n853 = Subtract(x=w1970, y=w1971) -> (x-y=w1969:u32)
              }
              n854 = while {
                tunnel: w1950 -> [w2097]
                tunnel: w1948 -> [w2091]
                tunnel: [w2094] -> _
                tunnel: [w2096] -> w1951
                i -> [w2098]
                stop <- w2094 stop-if-true
                # "Slightly faster version to read data"
                # "Get and display data"
                n855 = Dequeue Element(queue=w2091, timeout in ms (-1)=5000) -> (queue out=w2096:refnum<queue>, element=w2093:cluster{"gain":dbl, bool, "wfm":i16[][]})  [unwired: 1 in, 2 out]
                n856 = Unbundle(w2093) -> ("gain"=w2088:dbl, w2089:bool, "wfm"=w2090:i16[][])
                n857 = case shown="False" w2089 {
                  tunnel: w2090 -> [w2099 w2101]
                  tunnel: [w2099 w2100] -> w2092
                  frame False {
                  }
                  frame True {
                    n858 = call "ReverseData.vi"("Array in"=w2101) -> ("Array out"=w2100:i16[][])
                  }
                }
                n859 = Increment(x=w2098) -> (x+1=w2087:i32)
                n860 = local write "Display index"(w2087) -> ()
                n861 = call "CurrentPlane.vi"("gain"=w2088, "bits A/D"=13, "Axis Vals"=w2097, "Frame"=w2087, "Data"=w2092) -> ("stop out"=w2094:bool)  [unwired: 5 in, 1 out]
                n862 = local write "stop out"(w2094) -> ()
              }
              n863 = global read "MotionGlobals.vi" "DigTimeOut"() -> (w1940)
              n864 = while {
                tunnel: w1926 -> [w2045]
                tunnel: w1960 -> [w2044]
                tunnel: w1925 -> [w2043]
                tunnel: w1929 -> [w2042]
                tunnel: [w2041] -> w1953
                tunnel: w1945 -> [w2039]
                shift-right: [w2037] -> _
                shift-left: w1941 -> [w2038]
                tunnel: [w2036] -> _
                tunnel: w1940 -> [w2035]
                tunnel: "0,1" -> [w2034]
                tunnel: w1924 -> [w2033]
                tunnel: w1920 -> [w2032]
                stop <- w2040 stop-if-true
                n865 = for {
                  tunnel: w2042 -> [w2059]
                  tunnel: w2045 -> [w2061] mode=indexing
                  tunnel: w2034 -> [w2060]
                  tunnel: w2044 -> [w2058]
                  tunnel: [w2054] -> _
                  tunnel: w2043 -> [w2053]
                  tunnel: [w2051] -> w2041
                  tunnel: w2039 -> [w2050]
                  tunnel: w2035 -> [w2049]
                  tunnel: w2033 -> [w2047]
                  tunnel: w2032 -> [w2046]
                  i -> [w2048]
                  # "Read data"
                  n866 = case shown="1, Default" w2048 {
                    tunnel: w2061 -> [w2068 w2077]
                    tunnel: w2060 -> [w2066 w2076]
                    tunnel: w2059 -> [w2069 w2082]
                    tunnel: [w2070 w2081] -> w2057
                    tunnel: [w2063 w2075] -> w2056
                    tunnel: [w2071 w2080] -> w2054
                    tunnel: w2053 -> [w2072 _]
                    tunnel: [w2067 _] -> w2052
                    tunnel: w2050 -> [w2065 _]
                    tunnel: w2049 -> [_ w2078]
                    tunnel: w2047 -> [w2062 _]
                    tunnel: w2046 -> [_ w2073]
                    frame 0 {
                      # "Read files and queue it up."
                      n867 = call <instrlib>:"niScope Initiate Acquisition.vi"("instrument handle"=w2072) -> ("error out"=w2064:errorcluster)  [unwired: 2 in, 12 out]
                      n868 = call "Rapid Read_NI.vi"("Channel"=w2066, "lines per plane"=w2062, "error in"=w2064, "rf points per line"=w2069, "Motion Board ID"=w2065, "NI Card"=w2068) -> ("error out"=w2071:errorcluster, "Reverse?"=w2067:bool, "Array"=w2063:i8[][], "dig gain"=w2070:dbl)  [unwired: 2 in]
                    }
                    frame 1, Default {
                      n869 = property class="niScope"(reference=w2077, "Fetch Record Number"=0 ("Fetch:Fetch Record Number"), "Fetch Number of Records"=w2073) -> (reference out=w2083:refnum<k15>, error out=w2079:errorcluster)  [unwired: 1 in]
                      n870 = call-poly <instrlib>:"niScope Fetch (poly).vi"("timeout"=w2078, "error in"=w2079, "numSamples"=w2082, "channels"=w2076, "instrument handle"=w2083) -> ("error out"=w2080:errorcluster, "wfm"=w2075:i8[][], "wfm info"=w2085:T14)  [unwired: 4 out]
                      n871 = Index Array(array=w2085) -> (element=w2084:T15)  [unwired: 1 in]
                      n872 = Unbundle By Name(w2084) -> ("gain"=w2081:dbl)
                    }
                  }
                  n873 = local write "Read Data index"(w2048) -> ()
                  n874 = Bundle("gain"=w2057, "wfm"=w2056, "Reverse?"=w2052, w2048) -> (w2055:T16)  [unwired: 1 in]
                  n875 = Enqueue Element(queue=w2058, element=w2055) -> (queue out=w2051:refnum<queue>)  [unwired: 2 in, 2 out]
                }
                n876 = local read "stop out"() -> (w2040:bool)
                n877 = Tick Count (ms)() -> (millisecond timer value=w2037:u32)
                n878 = Subtract(x=w2037, y=w2038) -> (x-y=w2036:u32)
              }
              n879 = Release Queue(queue=w1953, force destroy? (F)=w1952) -> ()  [unwired: 1 in, 3 out]
              n880 = Release Queue(queue=w1951, force destroy? (F)=w1952) -> ()  [unwired: 1 in, 3 out]
              n881 = Delete Data Value Reference(data value reference=w1928) -> ()  [unwired: 1 in, 2 out]
            }
          }
        }
      }
    }
    frame #6 {
      n882 = case shown="2" w2104 {
        tunnel: w2103 -> [_ w2107]
        frame 0, Default {
        }
        frame 2 {
          n883 = for {
            tunnel: w2107 -> [w2110] mode=indexing
            n884 = call <vilib>:"DAQmx Stop Task.vi"("task/channels in"=w2110) -> ("task out"=w2109:refnum<k21>, "error out"=w2108:errorcluster)  [unwired: 13 in]
            n885 = call <vilib>:"DAQmx Clear Task.vi"("task in"=w2109, "error in"=w2108) -> ()  [unwired: 13 in, 1 out]
          }
        }
      }
      n886 = case shown="\"Hawaii\", Default" w2106 {
        frame "Hawaii", Default {
          # "turn off real time trig"
          n887 = call-poly <vilib>:"DAQmx Write.vi"("task/channels in"=refnum<k21> "DIO-L2 L3", "data"=bool[] [TRUE, FALSE]) -> ()  [unwired: 11 in, 3 out]
        }
        frame "UHI Allen" {
        }
      }
      n888 = local write "stop out"(FALSE ("stop out")) -> ()
      n889 = local write "Save Raw"(FALSE ("Save Raw")) -> ()
    }
  }
  n890 = case shown="0, Default" w38 {
    tunnel: w42 -> [w2114 w2119]
    tunnel: w41 -> [_ w2118]
    tunnel: w40 -> [w2113 w2117]
    tunnel: [w2114 w2116] -> w20
    tunnel: [w2113 w2115] -> w19
    frame 1, 8 {
    }
    frame 0, Default {
      n891 = call <vilib>:"Stop Program.flx"("error in (no error)"=w2117, "Program (1)"=w2118, "Board ID"=w2119) -> ("error out"=w2115:errorcluster, "Bd ID Out"=w2116:T2)  [unwired: 4 out]
    }
  }
  n892 = case shown="True" "return to start" {
    tunnel: w43 -> [_ w2127]
    tunnel: w39 -> [_ w2135]
    tunnel: w20 -> [w2121 w2126]
    tunnel: w19 -> [w2120 w2125]
    tunnel: [w2121 w2134] -> w18
    tunnel: w32 -> [_ w2133]
    tunnel: w30 -> [_ w2132]
    tunnel: [w2120 w2131] -> w29
    frame False {
    }
    frame True {
      n893 = call "MoveMotor.vi"("error in (no error)"=w2125, "Target Position (0)"=w2135, "Axis or Vector Space"=w2127, "Motion Bd ID"=w2126) -> ("error out"=w2123:errorcluster, "Resource Output"=w2122:u16, "Bd ID Out"=w2124:u8)  [unwired: 1 in, 4 out]
      n894 = call "Load Acceleration/Deceleration.flx"("Acceleration (100000)"=w2132, "error in (no error)"=w2123, "Axis or Vector Space"=w2122, "Board ID"=w2124) -> ("error out"=w2130:errorcluster, "Resource Output"=w2128:T18, "Bd ID Out"=w2129:T2)  [unwired: 1 in, 2 out]
      n895 = call <vilib>:"Load Velocity.flx"("Velocity (10000)"=w2133, "error in (no error)"=w2130, "Axis or Vector Space"=w2128, "Board ID"=w2129) -> ("error out"=w2131:errorcluster, "Bd ID Out"=w2134:T2)  [unwired: 4 out]
    }
  }
  "error out" <- w29
  n896 = flat-sequence {
    tunnel: w18 -> [w2136]
    frame #0 {
      "Bd ID Out" <- w2136
    }
    frame #1 {
      n897 = Wait (ms)(milliseconds to wait=u32 10) -> ()  [unwired: 1 out]
    }
  }
